vi "Autonomous Independent.vi"() -> ()   [LabVIEW 2017]
doc: "This VI is called when autonomous begins, and will automatically be terminated when autonomous ends. You can carry out timed or sensor driven robot movement independently without needing to return to the caller."
uses:
  CommandTypes/LiftCommands.ctl
  CommandTypes/AutoCommands.ctl
  <vilib>/Platform/TimedLoop/XDataNode/timing_clust.ctl
  <vilib>/Platform/TimedLoop/XDataNode/nitl_modes.ctl
  <vilib>/Platform/TimedLoop/XDataNode/wakeup.ctl
  <userlib>/836-Library/Drive/Drive_Code_V2/Drive_Code_Support/SensorTypedefs/Sensor_Cluster.ctl
  <userlib>/836-Library/Drive/Drive_Code_V2/Drive_Code_Support/SensorTypedefs/Camera_Cluster.ctl
  <vilib>/Rock Robotics/WPI/RobotDrive/WPI_RobotDriveDevRef.ctl
  <vilib>/Rock Robotics/WPI/MotorControl/WPI_MotorControlDeviceRef.ctl
  <vilib>/Rock Robotics/WPI/MotorControl/WPI_MotorControlType.ctl
  <vilib>/Rock Robotics/SystemInterfaces/DIO/FPGA_DIOPWMChannel.ctl
  <vilib>/Rock Robotics/WPI/PWM/WPI_PWMDeadband.ctl
  <vilib>/Rock Robotics/SystemInterfaces/DIO/FPGA_DIOChannel.ctl
  <userlib>/836-Library/Drive/Drive_Code_V2/Drive_Code_Support/DriveTrains/Drive_Trains.ctl
  <userlib>/836-Library/Drive/Drive_Code_V2/Drive_Code_Support/Command_Sends/Drive_Code_Command_Type.ctl
  <userlib>/836-Library/Drive/Drive_Code_V2/Drive_Code_Support/Command_Sends/Drive_Code_Command_List.ctl
  <userlib>/836-Library/Drive/Drive_Code_V2/Drive_Code_Support/PidClusters/PidInversions.ctl
  <userlib>/836-Library/Drive/Drive_Code_V2/Drive_Code_Support/PidClusters/DrivePidInputs.ctl
  <userlib>/836-Library/Drive/Drive_Code_V2/Drive_Code_Support/PidClusters/PidInputs.ctl
  <userlib>/836-Library/Drive/Drive_Code_V2/Drive_Code_Support/Command_Sends/Command_Tolerances.ctl
  <userlib>/836-Library/Drive/Drive_Code_V2/Drive_Code_Support/Command_Sends/Command_Tolerance_Info.ctl
  <userlib>/836-Library/Drive/Drive_Code_V2/Drive_Code_Support/CmdFinishedTypes.ctl
  CommandTypes/DriveCommands.ctl
  CommandTypes/IntakeCommands.ctl
  <vilib>/Rock Robotics/Network Tables/NT Read Number.vi
  <vilib>/Rock Robotics/Network Tables/NT Read Boolean.vi
  <vilib>/addons/control/pid/pid.llb/PID (DBL).vi
  <userlib>/836-Library/Drive/Drive_Code_V2/Drive_Code_Support/Command_Sends/Drive_Cmd_Cheesey_Drive.vi
  <userlib>/836-Library/Drive/Drive_Code_V2/Drive_Code_Support/Command_Sends/Drive_Cmd_Do_Nothing.vi
  <userlib>/836-Library/Drive/Drive_Code_V2/Drive_Code_Support/Command_Sends/Drive_Cmd_Drive_Distance.vi
  <vilib>/platform/TimedLoop/XDataNode/XDataNode.xnode
  <vilib>/Platform/TimedLoop/XDataNode/XDNodeRunTimeDep.lvlib
  <vilib>/addons/control/pid/NI_PID_pid.lvlib
  <userlib>/836-Library/Drive/Drive_Code_V2/Drive_Code_Support/Command_Sends/Drive_Cmd_Turn.vi
panel:
  in  "Y Points":dbl[](array[numeric])=[45.0, 40.0, 40.0, 45.0, 70.0]
  in  "X Points":dbl[](array[numeric])=[20.0, 50.0, 100.0, 200.0, 266.0]
  out "Throttle Cmd":dbl(graph)=-0.2211335616573206
  out "Steer Cmd":dbl(graph)=0.4174203899708857
  in  "Throttle Feed Fwd":dbl=0.28
  in  "Pid Setpoints":i32=500
  in  "Limit of Orientation Change":dbl=15.0 format="%#_13g"
  in  "Absolute Theta Final":dbl
  in  "Amount of Time (s)":dbl=4.0
  out "Steer Response":cluster{"setpoint":dbl, dbl}(graph)={"setpoint"=-0.6332041750032447, -21.50422367354753}
  in  "Steer Limit":cluster{"output high":dbl, "output low":dbl}={"output high"=0.5, "output low"=-0.5} {"output low" format="%.2f"; "output high" format="%.2f"}
  in  "Steer Gains":T1={"proportional gain (Kc)"=0.02, "integral time (Ti, min)"=0.0, "derivative time (Td, min)"=0.0} {"derivative time (Td, min)" format="%.3f"; "integral time (Ti, min)" format="%.3f"; "proportional gain (Kc)" format="%.3f"}
  out "Arc Response":cluster{"setpoint":dbl, dbl}(graph)={"setpoint"=251.75033529143298, 253.22199624999996}
  in  "Speed Limit":cluster{"output high":dbl, "output low":dbl}={"output high"=1.0, "output low"=-1.0} {"output low" format="%.2f"; "output high" format="%.2f"}
  in  "Speed Gains":T1={"proportional gain (Kc)"=0.04, "integral time (Ti, min)"=0.0, "derivative time (Td, min)"=0.0} {"derivative time (Td, min)" format="%.3f"; "integral time (Ti, min)" format="%.3f"; "proportional gain (Kc)" format="%.3f"}
  out "Auto Path Graph":cluster{"X":dbl, "Y":dbl}[](graph)=[{"X"=0.0, "Y"=0.0}, {"X"=0.29962072558749825, "Y"=0.0007367430518598614}, {"X"=0.5972966123215261, "Y"=0.0029335432231455886}, {"X"=0.8930518323738127, "Y"=0.0065702570374162475}, {"X"=1.1869105579160868, "Y"=0.011626741018230904}, {"X"=1.4788969611200782, "Y"=0.018082851689148624}, {"X"=1.7690352141575154, "Y"=0.025918445573728487}, {"X"=2.057349489200128, "Y"=0.035113379195529544}, {"X"=2.343863958419645, "Y"=0.04564750907811086}, {"X"=2.628602793987795, "Y"=0.057500691745031515}, {"X"=2.9115901680763074, "Y"=0.07065278371985056}, {"X"=3.192850252856912, "Y"=0.08508364152612709}, {"X"=3.4724072205013368, "Y"=0.10077312168742014}, {"X"=3.750285243181312, "Y"=0.1177010807272888}, {"X"=4.026508493068566, "Y"=0.13584737516929213}, {"X"=4.3011011423348275, "Y"=0.15519186153698913}, {"X"=4.574087363151827, "Y"=0.175714396353939}, {"X"=4.845491327691294, "Y"=0.19739483614370076}, {"X"=5.115337208124954, "Y"=0.2202130374298334}, {"X"=5.38364917662454, "Y"=0.24414885673589606}, {"X"=5.650451405361779, "Y"=0.2691821505854477}, {"X"=5.915768066508401, "Y"=0.2952927755020476}, {"X"=6.179623332236137, "Y"=0.3224605880092547}, {"X"=6.442041374716712, "Y"=0.35066544463062793}, {"X"=6.703046366121857, "Y"=0.37988720188972663}, {"X"=6.962662478623301, "Y"=0.4101057163101096}, {"X"=7.2209138843927745, "Y"=0.4413008444153362}, {"X"=7.477824755602007, "Y"=0.4734524427289652}, {"X"=7.733419264422724, "Y"=0.5065403677745559}, {"X"=7.987721583026658, "Y"=0.5405444760756672}, {"X"=8.240755883585535, "Y"=0.5754446241558583}, {"X"=8.492546338271088, "Y"=0.6112206685386881}, {"X"=8.743117119255043, "Y"=0.6478524657477159}, {"X"=8.992492398709132, "Y"=0.6853198723065006}, {"X"=9.24069634880508, "Y"=0.7236027447386013}, {"X"=9.48775314171462, "Y"=0.7626809395675768}, {"X"=9.73368694960948, "Y"=0.8025343133169868}, {"X"=9.978521944661388, "Y"=0.8431427225103897}, {"X"=10.222282299042075, "Y"=0.8844860236713451}, {"X"=10.464992184923267, "Y"=0.9265440733234118}, {"X"=10.706675774476695, "Y"=0.9692967279901487}, {"X"=10.94735723987409, "Y"=1.0127238441951152}, {"X"=11.187060753287179, "Y"=1.0568052784618704}, {"X"=11.425810486887691, "Y"=1.1015208873139732}, {"X"=11.663630612847356, "Y"=1.1468505272749825}, {"X"=11.900545303337903, "Y"=1.1927740548684576}, {"X"=12.13657873053106, "Y"=1.2392713266179574}, {"X"=12.371755066598556, "Y"=1.286322199047041}, {"X"=12.606098483712124, "Y"=1.333906528679268}, {"X"=12.839633154043486, "Y"=1.3820041720381968}, {"X"=13.072383249764378, "Y"=1.4305949856473863}, {"X"=13.304372943046527, "Y"=1.4796588260303962}, {"X"=13.535626406061661, "Y"=1.5291755497107853}, {"X"=13.76616781098151, "Y"=1.5791250132121126}, {"X"=13.996021329977804, "Y"=1.6294870730579374}, {"X"=14.225211135222267, "Y"=1.6802415857718185}, {"X"=14.453761398886636, "Y"=1.7313684078773153}, {"X"=14.681696293142636, "Y"=1.7828473958979865}, {"X"=14.909039990161995, "Y"=1.8346584063573912}, {"X"=15.135816662116438, "Y"=1.886781295779088}, {"X"=15.362050481177707, "Y"=1.9391959206866372}, {"X"=15.587765619517521, "Y"=1.9918821376035971}, {"X"=15.812986249307613, "Y"=2.0448198030535267}, {"X"=16.03773654271971, "Y"=2.097988773559986}, {"X"=16.26204067192554, "Y"=2.1513689056465326}, {"X"=16.485922809096838, "Y"=2.2049400558367265}, {"X"=16.709407126405328, "Y"=2.2586820806541263}, {"X"=16.93251779602274, "Y"=2.3125748366222916}, {"X"=17.155278990120802, "Y"=2.3665981802647806}, {"X"=17.377714880871245, "Y"=2.420731968105154}, {"X"=17.599849640445797, "Y"=2.474956056666968}, {"X"=17.82170744101619, "Y"=2.5292503024737854}, {"X"=18.04331245475415, "Y"=2.5835945620491625}, {"X"=18.26468885383141, "Y"=2.6379686919166594}, {"X"=18.48586081041969, "Y"=2.692352548599834}, {"X"=18.70685249669073, "Y"=2.7467259886222477}, {"X"=18.927688084816253, "Y"=2.8010688685074574}, {"X"=19.14839174696799, "Y"=2.855361044779024}, {"X"=19.36898765531767, "Y"=2.9095823739605042}, {"X"=19.589499982037022, "Y"=2.9637127125754597}, {"X"=19.809952899297773, "Y"=3.0177319171474464}, {"X"=20.030370579271654, "Y"=3.071619844200027}, {"X"=20.250777194130396, "Y"=3.125356350256758}, {"X"=20.471196916045724, "Y"=3.1789212918411995}, {"X"=20.691653917189374, "Y"=3.23229452547691}, {"X"=20.912172369733067, "Y"=3.28545590768745}, {"X"=21.132776445848535, "Y"=3.3383852949963764}, {"X"=21.35349031770751, "Y"=3.39106254392725}, {"X"=21.57433815748172, "Y"=3.4434675110036284}, {"X"=21.795344137342887, "Y"=3.495580052749072}, {"X"=22.01653242946275, "Y"=3.5473800256871395}, {"X"=22.237927206013033, "Y"=3.5988472863413894}, {"X"=22.459552639165466, "Y"=3.6499616912353807}, {"X"=22.68143290109178, "Y"=3.700703096892674}, {"X"=22.903592163963708, "Y"=3.7510513598368265}, {"X"=23.126054599952965, "Y"=3.800986336591399}, {"X"=23.34884438123129, "Y"=3.850487883679948}, {"X"=23.571985679970414, "Y"=3.8995358576260357}, {"X"=23.795502668342063, "Y"=3.9481101149532196}, {"X"=24.019419518517964, "Y"=3.9961905121850583}, {"X"=24.24376040266985, "Y"=4.043756905845111}, {"X"=24.468549492969448, "Y"=4.090789152456939}, {"X"=24.693810961588486, "Y"=4.137267108544098}, {"X"=24.9195689806987, "Y"=4.183170630630149}, {"X"=25.145847722471807, "Y"=4.22847957523865}, {"X"=25.37267135907955, "Y"=4.273173798893161}, {"X"=25.600064062693644, "Y"=4.317233158117241}, {"X"=25.828050005485824, "Y"=4.360637509434449}, {"X"=26.05665335962783, "Y"=4.403366709368345}, {"X"=26.28589829729137, "Y"=4.445400614442485}, {"X"=26.515808990648196, "Y"=4.486719081180431}, {"X"=26.746409611870018, "Y"=4.527301966105741}, {"X"=26.977724333128574, "Y"=4.567129125741975}, {"X"=27.209777326595592, "Y"=4.60618041661269}, {"X"=27.442592764442804, "Y"=4.644435695241447}, {"X"=27.676194818841932, "Y"=4.681874818151805}, {"X"=27.910607661964715, "Y"=4.718477641867323}, {"X"=28.145855465982866, "Y"=4.754224022911557}, {"X"=28.38196240306813, "Y"=4.7890938178080695}, {"X"=28.618952645392234, "Y"=4.82306688308042}, {"X"=28.8568503651269, "Y"=4.856123075252166}, {"X"=29.095679734443863, "Y"=4.888242250846866}, {"X"=29.335464925514845, "Y"=4.919404266388079}, {"X"=29.576230110511585, "Y"=4.949588978399366}, {"X"=29.817999461605805, "Y"=4.978776243404285}, {"X"=30.060797180862526, "Y"=5.006946007031386}, {"X"=30.30465108743448, "Y"=5.034088996613002}, {"X"=30.549596025396845, "Y"=5.06021687915411}, {"X"=30.795667645943535, "Y"=5.085343727494415}, {"X"=31.042901600268472, "Y"=5.109483614473622}, {"X"=31.291333539565585, "Y"=5.132650612931439}, {"X"=31.54099911502878, "Y"=5.154858795707567}, {"X"=31.79193397785199, "Y"=5.176122235641715}, {"X"=32.04417377922912, "Y"=5.196455005573586}, {"X"=32.29775417035411, "Y"=5.215871178342887}, {"X"=32.55271080242086, "Y"=5.234384826789322}, {"X"=32.809079326623305, "Y"=5.2520100237525975}, {"X"=33.06689539415536, "Y"=5.268760842072417}, {"X"=33.326194656210944, "Y"=5.284651354588488}, {"X"=33.58701276398397, "Y"=5.299695634140513}, {"X"=33.84938536866837, "Y"=5.3139077535682}, {"X"=34.11334812145807, "Y"=5.327301785711254}, {"X"=34.37893667354697, "Y"=5.339891803409379}, {"X"=34.646186676129005, "Y"=5.351691879502281}, {"X"=34.91513378039809, "Y"=5.362716086829666}, {"X"=35.18581363754814, "Y"=5.372978498231237}, {"X"=35.45826189877308, "Y"=5.382493186546703}, {"X"=35.73251421526684, "Y"=5.391274224615765}, {"X"=36.00860623822332, "Y"=5.399335685278132}, {"X"=36.28657361883646, "Y"=5.4066916413735076}, {"X"=36.56645200830016, "Y"=5.413356165741597}, {"X"=36.84827705780836, "Y"=5.419343331222105}, {"X"=37.132084418554975, "Y"=5.424667210654739}, {"X"=37.41790974173391, "Y"=5.429341876879203}, {"X"=37.70578867853911, "Y"=5.433381402735202}, {"X"=37.995756880164464, "Y"=5.436799861062442}, {"X"=38.287849997803924, "Y"=5.4396113247006275}, {"X"=38.58210368265139, "Y"=5.441829866489465}, {"X"=38.87855358590079, "Y"=5.443469559268658}, {"X"=39.177235358746046, "Y"=5.4445444758779145}, {"X"=39.47818465238106, "Y"=5.445068689156937}, {"X"=39.781437117999786, "Y"=5.4450562719454325}, {"X"=40.08702840679611, "Y"=5.444521297083106}, {"X"=40.39499416996397, "Y"=5.443477837409661}, {"X"=40.705370058697284, "Y"=5.441939965764806}, {"X"=41.018191724189975, "Y"=5.439921754988245}, {"X"=41.33349481763595, "Y"=5.437437277919683}, {"X"=41.651314990229146, "Y"=5.4345006073988245}, {"X"=41.97168789316346, "Y"=5.431125816265377}, {"X"=42.29464917763285, "Y"=5.427326977359043}, {"X"=42.620234494831195, "Y"=5.42311816351953}, {"X"=42.94847949595244, "Y"=5.418513447586543}, {"X"=43.279419832190506, "Y"=5.413526902399787}, {"X"=43.613091154739294, "Y"=5.408172600798967}, {"X"=43.949529114792746, "Y"=5.402464615623788}, {"X"=44.28876936354476, "Y"=5.396417019713956}, {"X"=44.63084755218928, "Y"=5.390043885909177}, {"X"=44.9757993319202, "Y"=5.383359287049155}, {"X"=45.32366035393147, "Y"=5.376377295973596}, {"X"=45.67446626941699, "Y"=5.3691119855222045}, {"X"=46.02825272957068, "Y"=5.361577428534686}, {"X"=46.38505538558647, "Y"=5.3537876978507475}, {"X"=46.74490988865826, "Y"=5.345756866310093}, {"X"=47.107851889980005, "Y"=5.337499006752427}, {"X"=47.47391704074559, "Y"=5.329028192017456}, {"X"=47.84314099214896, "Y"=5.320358494944885}, {"X"=48.21555939538402, "Y"=5.31150398837442}, {"X"=48.5912079016447, "Y"=5.3024787451457644}, {"X"=48.97012216212491, "Y"=5.293296838098625}, {"X"=49.352337828018584, "Y"=5.283972340072706}, {"X"=49.73789055051962, "Y"=5.2745193239077155}, {"X"=50.126815980821966, "Y"=5.264951862443355}, {"X"=50.519149770119526, "Y"=5.255284028519333}, {"X"=50.914927569606206, "Y"=5.245529894975353}, {"X"=51.31418503047596, "Y"=5.235703534651121}, {"X"=51.71695780392268, "Y"=5.225819020386341}, {"X"=52.1232815411403, "Y"=5.21589042502072}, {"X"=52.53319189332274, "Y"=5.205931821393963}, {"X"=52.946724511663916, "Y"=5.195957282345774}, {"X"=53.36391504735774, "Y"=5.185980880715861}, {"X"=53.78479915159815, "Y"=5.176016689343926}, {"X"=54.20941247557906, "Y"=5.166078781069676}, {"X"=54.63779067049438, "Y"=5.156181228732817}, {"X"=55.06996938753802, "Y"=5.1463381051730535}, {"X"=55.50598427790395, "Y"=5.136563483230091}, {"X"=55.94587099278605, "Y"=5.1268714357436345}, {"X"=56.38966518337824, "Y"=5.117276035553388}, {"X"=56.83740250087444, "Y"=5.10779135549906}, {"X"=57.2891185964686, "Y"=5.098431468420354}, {"X"=57.744849121354605, "Y"=5.089210447156975}, {"X"=58.204629726726395, "Y"=5.080142364548628}, {"X"=58.66849606377785, "Y"=5.07124129343502}, {"X"=59.136483783702964, "Y"=5.062521306655855}, {"X"=59.6086285376956, "Y"=5.0539964770508385}, {"X"=60.08496597694969, "Y"=5.045680877459676}, {"X"=60.56553175265917, "Y"=5.0375885807220735}, {"X"=61.050361516017944, "Y"=5.029733659677735}, {"X"=61.53949091821995, "Y"=5.022130187166366}, {"X"=62.03295561045906, "Y"=5.014792236027673}, {"X"=62.53079124392925, "Y"=5.007733879101359}, {"X"=63.03303346982443, "Y"=5.000969189227131}, {"X"=63.53971793933851, "Y"=4.9945122392446955}, {"X"=64.05088030366538, "Y"=4.9883771019937555}, {"X"=64.56655621399901, "Y"=4.982577850314018}, {"X"=65.08678132153331, "Y"=4.977128557045186}, {"X"=65.61159127746217, "Y"=4.972043295026968}, {"X"=66.14102173297954, "Y"=4.967336137099067}, {"X"=66.67510833927932, "Y"=4.963021156101189}, {"X"=67.21388674755546, "Y"=4.959112424873039}, {"X"=67.75739260900183, "Y"=4.955624016254323}, {"X"=68.3056615748124, "Y"=4.952570003084746}, {"X"=68.85872929618108, "Y"=4.949964458204013}, {"X"=69.41663142430178, "Y"=4.947821454451829}, {"X"=69.9794036103684, "Y"=4.946155064667901}, {"X"=70.54708150557488, "Y"=4.9449793616919315}, {"X"=71.11970076111515, "Y"=4.944308418363629}, {"X"=71.69729702818313, "Y"=4.944156307522697}, {"X"=72.27990595797272, "Y"=4.94453710200884}, {"X"=72.86756320167787, "Y"=4.945464874661765}, {"X"=73.46030441049247, "Y"=4.946953698321177}, {"X"=74.05816523561043, "Y"=4.949017645826781}, {"X"=74.66118132822572, "Y"=4.951670790018282}, {"X"=75.26938833953223, "Y"=4.954927203735385}, {"X"=75.88282192072388, "Y"=4.958800959817797}, {"X"=76.50151772299456, "Y"=4.963306131105221}, {"X"=77.12551139753825, "Y"=4.968456790437365}, {"X"=77.75483859554886, "Y"=4.974267010653931}, {"X"=78.38953496822026, "Y"=4.980750864594628}, {"X"=79.02963616674641, "Y"=4.987922425099159}, {"X"=79.67517784232123, "Y"=4.995795765007229}, {"X"=80.32619336045194, "Y"=5.004383910893502}, {"X"=80.98266351585136, "Y"=5.013675825236637}, {"X"=81.64451653243808, "Y"=5.0236364064193015}, {"X"=82.3116783484439, "Y"=5.034229506559112}, {"X"=82.98407490210067, "Y"=5.045418977773689}, {"X"=83.66163213164016, "Y"=5.057168672180652}, {"X"=84.34427597529427, "Y"=5.069442441897622}, {"X"=85.03193237129477, "Y"=5.082204139042218}, {"X"=85.72452725787349, "Y"=5.0954176157320585}, {"X"=86.42198657326229, "Y"=5.109046724084765}, {"X"=87.12423625569298, "Y"=5.123055316217956}, {"X"=87.83120224339737, "Y"=5.137407244249251}, {"X"=88.54281047460726, "Y"=5.15206636029627}, {"X"=89.25898688755456, "Y"=5.166996516476634}, {"X"=89.97965742047104, "Y"=5.182161564907961}, {"X"=90.70474801158852, "Y"=5.197525357707872}, {"X"=91.43418459913882, "Y"=5.213051746993985}, {"X"=92.1678931213538, "Y"=5.228704584883921}, {"X"=92.90579951646528, "Y"=5.2444477234953}, {"X"=93.64782972270503, "Y"=5.26024501494574}, {"X"=94.39390967830495, "Y"=5.276060311352863}, {"X"=95.14396532149684, "Y"=5.291857464834287}, {"X"=95.89792259051252, "Y"=5.307600327507632}, {"X"=96.65570742358378, "Y"=5.323252751490518}, {"X"=97.4172457589425, "Y"=5.338778588900565}, {"X"=98.1824635348205, "Y"=5.354141691855392}, {"X"=98.95128668944957, "Y"=5.369305912472619}, {"X"=99.72364116106155, "Y"=5.384235102869865}, {"X"=100.49945288788828, "Y"=5.398893115164751}, {"X"=101.2786478081616, "Y"=5.413243801474897}, {"X"=102.06115186011326, "Y"=5.427251013917919}, {"X"=102.84689098197518, "Y"=5.4408786046114415}, {"X"=103.63579111197913, "Y"=5.454090425673082}, {"X"=104.42777818835697, "Y"=5.466850329220461}, {"X"=105.22277814934046, "Y"=5.479122167371195}, {"X"=106.0207169331615, "Y"=5.490869792242909}, {"X"=106.82152047805188, "Y"=5.502057055953219}, {"X"=107.62511472224344, "Y"=5.512647810619745}, {"X"=108.43142560396794, "Y"=5.522605908360108}, {"X"=109.24037906145732, "Y"=5.531895201291926}, {"X"=110.05190103294333, "Y"=5.540479541532821}, {"X"=110.86591745665778, "Y"=5.54832278120041}, {"X"=111.68235427083256, "Y"=5.555388772412315}, {"X"=112.50113741369947, "Y"=5.561641367286155}, {"X"=113.32219282349033, "Y"=5.567044417939549}, {"X"=114.1454464384369, "Y"=5.571561776490117}, {"X"=114.97082419677113, "Y"=5.5751572950554795}, {"X"=115.79825203672479, "Y"=5.577794825753255}, {"X"=116.62765589652966, "Y"=5.579438220701063}, {"X"=117.4589617144176, "Y"=5.5800513320165255}, {"X"=118.29209542862048, "Y"=5.57959801181726}, {"X"=119.12698297737006, "Y"=5.578042112220887}, {"X"=119.96355029889817, "Y"=5.575347485345026}, {"X"=120.8017233314367, "Y"=5.571477983307297}, {"X"=121.64142801321742, "Y"=5.566397458225318}, {"X"=122.48259028247216, "Y"=5.5600697622167115}, {"X"=123.32513607743273, "Y"=5.552458747399096}, {"X"=124.168991336331, "Y"=5.543528265890091}, {"X"=125.01408199739879, "Y"=5.533242169807315}, {"X"=125.8603339988679, "Y"=5.521564311268389}, {"X"=126.70767327897012, "Y"=5.508458542390934}, {"X"=127.55602577593737, "Y"=5.4938887152925675}, {"X"=128.4053174280014, "Y"=5.47781868209091}, {"X"=129.25547417339405, "Y"=5.460212294903582}, {"X"=130.10642195034717, "Y"=5.441033405848201}, {"X"=130.9580866970926, "Y"=5.4202458670423885}, {"X"=131.8103943518621, "Y"=5.397813530603764}, {"X"=132.6632708528875, "Y"=5.373700248649947}, {"X"=133.51664213840073, "Y"=5.347869873298557}, {"X"=134.3704341466335, "Y"=5.320286256667213}, {"X"=135.22457281581768, "Y"=5.290913250873538}, {"X"=136.0789840841851, "Y"=5.259714708035148}, {"X"=136.9335938899676, "Y"=5.226654480269662}, {"X"=137.78832817139696, "Y"=5.191696419694703}, {"X"=138.643112866705, "Y"=5.154804378427891}, {"X"=139.4978739141236, "Y"=5.115942208586842}, {"X"=140.35253725188457, "Y"=5.075073762289178}, {"X"=141.20702881821973, "Y"=5.0321628916525185}, {"X"=142.06127455136087, "Y"=4.9871734487944845}, {"X"=142.91520038953985, "Y"=4.940069285832693}, {"X"=143.76873227098855, "Y"=4.890814254884764}, {"X"=144.62179613393863, "Y"=4.839372208068322}, {"X"=145.4743179166221, "Y"=4.785706997500979}, {"X"=146.3262235572707, "Y"=4.729782475300358}, {"X"=147.17743899411627, "Y"=4.671562493584082}, {"X"=148.0278901653906, "Y"=4.611010904469768}, {"X"=148.87750300932555, "Y"=4.548091560075034}, {"X"=149.72620346415295, "Y"=4.482768312517502}, {"X"=150.57391746810464, "Y"=4.41500501391479}, {"X"=151.42057095941237, "Y"=4.344765516384522}, {"X"=152.26608987630803, "Y"=4.272013672044311}, {"X"=153.11040015702346, "Y"=4.196713333011781}, {"X"=153.9534277397904, "Y"=4.118828351404554}, {"X"=154.79509856284076, "Y"=4.038322579340243}, {"X"=155.63533856440637, "Y"=3.955159868936471}, {"X"=156.474073682719, "Y"=3.8693040723108583}, {"X"=157.31122985601047, "Y"=3.7807190415810275}, {"X"=158.14673302251265, "Y"=3.689368628864591}, {"X"=158.98050912045738, "Y"=3.5952166862791737}, {"X"=159.81248408807642, "Y"=3.498227065942393}, {"X"=160.6425838636016, "Y"=3.3983636199718736}, {"X"=161.47073438526482, "Y"=3.295590200485228}, {"X"=162.29686159129787, "Y"=3.1898706596000785}, {"X"=163.12089141993252, "Y"=3.081168849434051}, {"X"=163.94274980940065, "Y"=2.969448622104754}, {"X"=164.76236269793412, "Y"=2.854673829729813}, {"X"=165.5796560237647, "Y"=2.7368083244268484}, {"X"=166.39455572512418, "Y"=2.615815958313483}, {"X"=167.20698774024447, "Y"=2.4916605835073273}, {"X"=168.01687800735735, "Y"=2.364306052126008}, {"X"=168.8241524646947, "Y"=2.233716216287141}, {"X"=169.6287370504882, "Y"=2.0998549281083543}, {"X"=170.43055770296985, "Y"=1.9626860397072563}, {"X"=171.22954036037137, "Y"=1.8221734032014707}, {"X"=172.0256109609246, "Y"=1.6782808707086256}, {"X"=172.81869544286138, "Y"=1.5309722943463262}, {"X"=173.60871974441358, "Y"=1.3802115262321992}, {"X"=174.395609803813, "Y"=1.225962418483865}, {"X"=175.17929155929136, "Y"=1.0681888232189483}, {"X"=175.9596909490806, "Y"=0.9068545925550575}, {"X"=176.73673391141256, "Y"=0.7419235786098177}, {"X"=177.51034638451898, "Y"=0.5733596335008491}, {"X"=178.28045430663173, "Y"=0.40112660934577704}, {"X"=179.04698361598264, "Y"=0.22518835826221117}, {"X"=179.80986025080355, "Y"=0.04550873236777253}, {"X"=180.5690154266411, "Y"=-0.1379399569945681}, {"X"=181.32442629122727, "Y"=-0.32511177189097307}, {"X"=182.0760936424828, "Y"=-0.5159228645258761}, {"X"=182.8240184737846, "Y"=-0.7102890737990789}, {"X"=183.5682017785096, "Y"=-0.9081262386103742}, {"X"=184.30864455003476, "Y"=-1.1093501978595812}, {"X"=185.04534778173695, "Y"=-1.3138767904464923}, {"X"=185.77831246699316, "Y"=-1.5216218552709098}, {"X"=186.50753959918018, "Y"=-1.7325012312326256}, {"X"=187.23303017167507, "Y"=-1.9464307572314596}, {"X"=187.95478517785472, "Y"=-2.163326272167204}, {"X"=188.67280561109595, "Y"=-2.383103614939652}, {"X"=189.3870924647758, "Y"=-2.6056786244486227}, {"X"=190.09764673227116, "Y"=-2.830967139593909}, {"X"=190.8044694069589, "Y"=-3.0588849992753127}, {"X"=191.50756148221598, "Y"=-3.289348042392625}, {"X"=192.20692395141933, "Y"=-3.522272107845667}, {"X"=192.90255780794587, "Y"=-3.7575730345342313}, {"X"=193.5944640451725, "Y"=-3.9951666613581187}, {"X"=194.28264365647613, "Y"=-4.234968827217121}, {"X"=194.9670976352337, "Y"=-4.47689537101106}, {"X"=195.64782697482215, "Y"=-4.720862131639728}, {"X"=196.32483266861834, "Y"=-4.966784948002913}, {"X"=196.99811570999924, "Y"=-5.214579659000441}, {"X"=197.6676770923418, "Y"=-5.464162103532102}, {"X"=198.33351780902285, "Y"=-5.715448120497686}, {"X"=198.99563885341936, "Y"=-5.968353548797018}, {"X"=199.65404121890828, "Y"=-6.222794227329887}, {"X"=200.3087258988665, "Y"=-6.478685994996095}, {"X"=200.95969388667095, "Y"=-6.735944690695444}, {"X"=201.6069461756985, "Y"=-6.994486153327736}, {"X"=202.2504837593261, "Y"=-7.254226221792747}, {"X"=202.89030763093075, "Y"=-7.5150807349903275}, {"X"=203.52641878388926, "Y"=-7.776965531820255}, {"X"=204.15881821157862, "Y"=-8.039796451182331}, {"X"=204.7875069073757, "Y"=-8.303489331976358}, {"X"=205.41248586465747, "Y"=-8.567960013102136}, {"X"=206.0337560768008, "Y"=-8.833124333459468}, {"X"=206.65131853718265, "Y"=-9.098898131948154}, {"X"=207.26517423917986, "Y"=-9.365197247467975}, {"X"=207.87532417616947, "Y"=-9.631937518918777}, {"X"=208.48176934152835, "Y"=-9.899034785200337}, {"X"=209.08451072863343, "Y"=-10.16640488521246}, {"X"=209.6835493308616, "Y"=-10.433963657854944}, {"X"=210.2788861415898, "Y"=-10.701626942027595}, {"X"=210.87052215419493, "Y"=-10.969310576630209}, {"X"=211.4584583620539, "Y"=-11.236930400562569}, {"X"=212.04269575854372, "Y"=-11.504402252724521}, {"X"=212.62323533704122, "Y"=-11.771641972015846}, {"X"=213.20007809092334, "Y"=-12.03856539733634}, {"X"=213.77322501356704, "Y"=-12.30508836758581}, {"X"=214.3426770983492, "Y"=-12.571126721664054}, {"X"=214.90843533864674, "Y"=-12.836596298470877}, {"X"=215.47050072783657, "Y"=-13.101412936906053}, {"X"=216.02887425929563, "Y"=-13.365492475869434}, {"X"=216.5835569264009, "Y"=-13.628750754260796}, {"X"=217.1345497225292, "Y"=-13.891103610979942}, {"X"=217.6818536410575, "Y"=-14.152466884926673}, {"X"=218.2254696753627, "Y"=-14.412756415000791}, {"X"=218.76539881882172, "Y"=-14.671888040102095}, {"X"=219.30164206481155, "Y"=-14.929777599130391}, {"X"=219.83420040670896, "Y"=-15.186340930985457}, {"X"=220.36307483789102, "Y"=-15.441493874567135}, {"X"=220.8882663517346, "Y"=-15.69515226877521}, {"X"=221.4097759416166, "Y"=-15.94723195250948}, {"X"=221.92760460091398, "Y"=-16.197648764669747}, {"X"=222.4417533230036, "Y"=-16.44631854415581}, {"X"=222.95222310126246, "Y"=-16.69315712986748}, {"X"=223.45901492906737, "Y"=-16.93808036070453}, {"X"=223.96212979979535, "Y"=-17.1810040755668}, {"X"=224.4615687068233, "Y"=-17.421844113354084}, {"X"=224.9573326435281, "Y"=-17.660516312966166}, {"X"=225.44942260328673, "Y"=-17.89693651330286}, {"X"=225.93783957947605, "Y"=-18.131020553263966}, {"X"=226.42258456547302, "Y"=-18.362684271749284}, {"X"=226.90365855465453, "Y"=-18.591843507658595}, {"X"=227.38106254039752, "Y"=-18.818414099891736}, {"X"=227.85479751607895, "Y"=-19.0423118873485}, {"X"=228.32486447507566, "Y"=-19.263452708928682}, {"X"=228.79126441076463, "Y"=-19.48175240353208}, {"X"=229.25399831652277, "Y"=-19.697126810058503}, {"X"=229.71306718572697, "Y"=-19.909491767407747}, {"X"=230.16847201175418, "Y"=-20.118763114479613}, {"X"=230.62021378798127, "Y"=-20.32485669017389}, {"X"=231.06829350778526, "Y"=-20.52768833339041}, {"X"=231.51271216454296, "Y"=-20.727173883028964}, {"X"=231.9534707516314, "Y"=-20.923229177989345}, {"X"=232.39057026242742, "Y"=-21.115770057171357}, {"X"=232.82401169030794, "Y"=-21.304712359474806}, {"X"=233.25379602864996, "Y"=-21.489971923799487}, {"X"=233.67992427083027, "Y"=-21.671464589045197}, {"X"=234.10239741022588, "Y"=-21.84910619411175}, {"X"=234.52121644021372, "Y"=-22.022812577898954}, {"X"=234.9363823541707, "Y"=-22.192499579306592}, {"X"=235.3478961454737, "Y"=-22.35808303723448}, {"X"=235.75575880749966, "Y"=-22.519478790582408}, {"X"=236.15997133362552, "Y"=-22.676602678250187}, {"X"=236.56053471722817, "Y"=-22.829370539137596}, {"X"=236.95744995168457, "Y"=-22.977698212144468}, {"X"=237.35071803037158, "Y"=-23.121501536170594}, {"X"=237.7403399466662, "Y"=-23.260696350115776}, {"X"=238.1263166939453, "Y"=-23.395198492879803}, {"X"=238.5086492655858, "Y"=-23.524923803362494}, {"X"=238.88733865496465, "Y"=-23.64978812046364}, {"X"=239.26238585545872, "Y"=-23.769707283083047}, {"X"=239.63379186044494, "Y"=-23.884597130120504}, {"X"=240.0015576633003, "Y"=-23.99437350047583}, {"X"=240.36568425740165, "Y"=-24.098952233048824}, {"X"=240.72617263612594, "Y"=-24.198249166739277}, {"X"=241.08302379285007, "Y"=-24.292180140447005}, {"X"=241.43623872095097, "Y"=-24.3806609930718}, {"X"=241.78581841380557, "Y"=-24.463607563513463}, {"X"=242.13176386479074, "Y"=-24.54093569067179}, {"X"=242.4740760672835, "Y"=-24.6125612134466}, {"X"=242.8127560146607, "Y"=-24.678399970737686}, {"X"=243.14780470029928, "Y"=-24.738367801444845}, {"X"=243.4792231175761, "Y"=-24.79238054446789}, {"X"=243.8070122598682, "Y"=-24.840354038706604}, {"X"=244.1311731205524, "Y"=-24.882204123060802}, {"X"=244.45170669300563, "Y"=-24.917846636430284}, {"X"=244.7686139706049, "Y"=-24.947197417714847}, {"X"=245.081895946727, "Y"=-24.9701723058143}, {"X"=245.39155361474897, "Y"=-24.98668713962844}, {"X"=245.69758796804766, "Y"=-24.99665775805707}, {"X"=246.0, "Y"=-24.999999999999993}]
  out "Init Heights Queue":T2[](array[typedef])
  out "Init Turns Queue":dbl[](array[numeric])
  out "Init Points Queue":cluster{"X Points":dbl[], "Y Points":dbl[]}[](array[cluster])
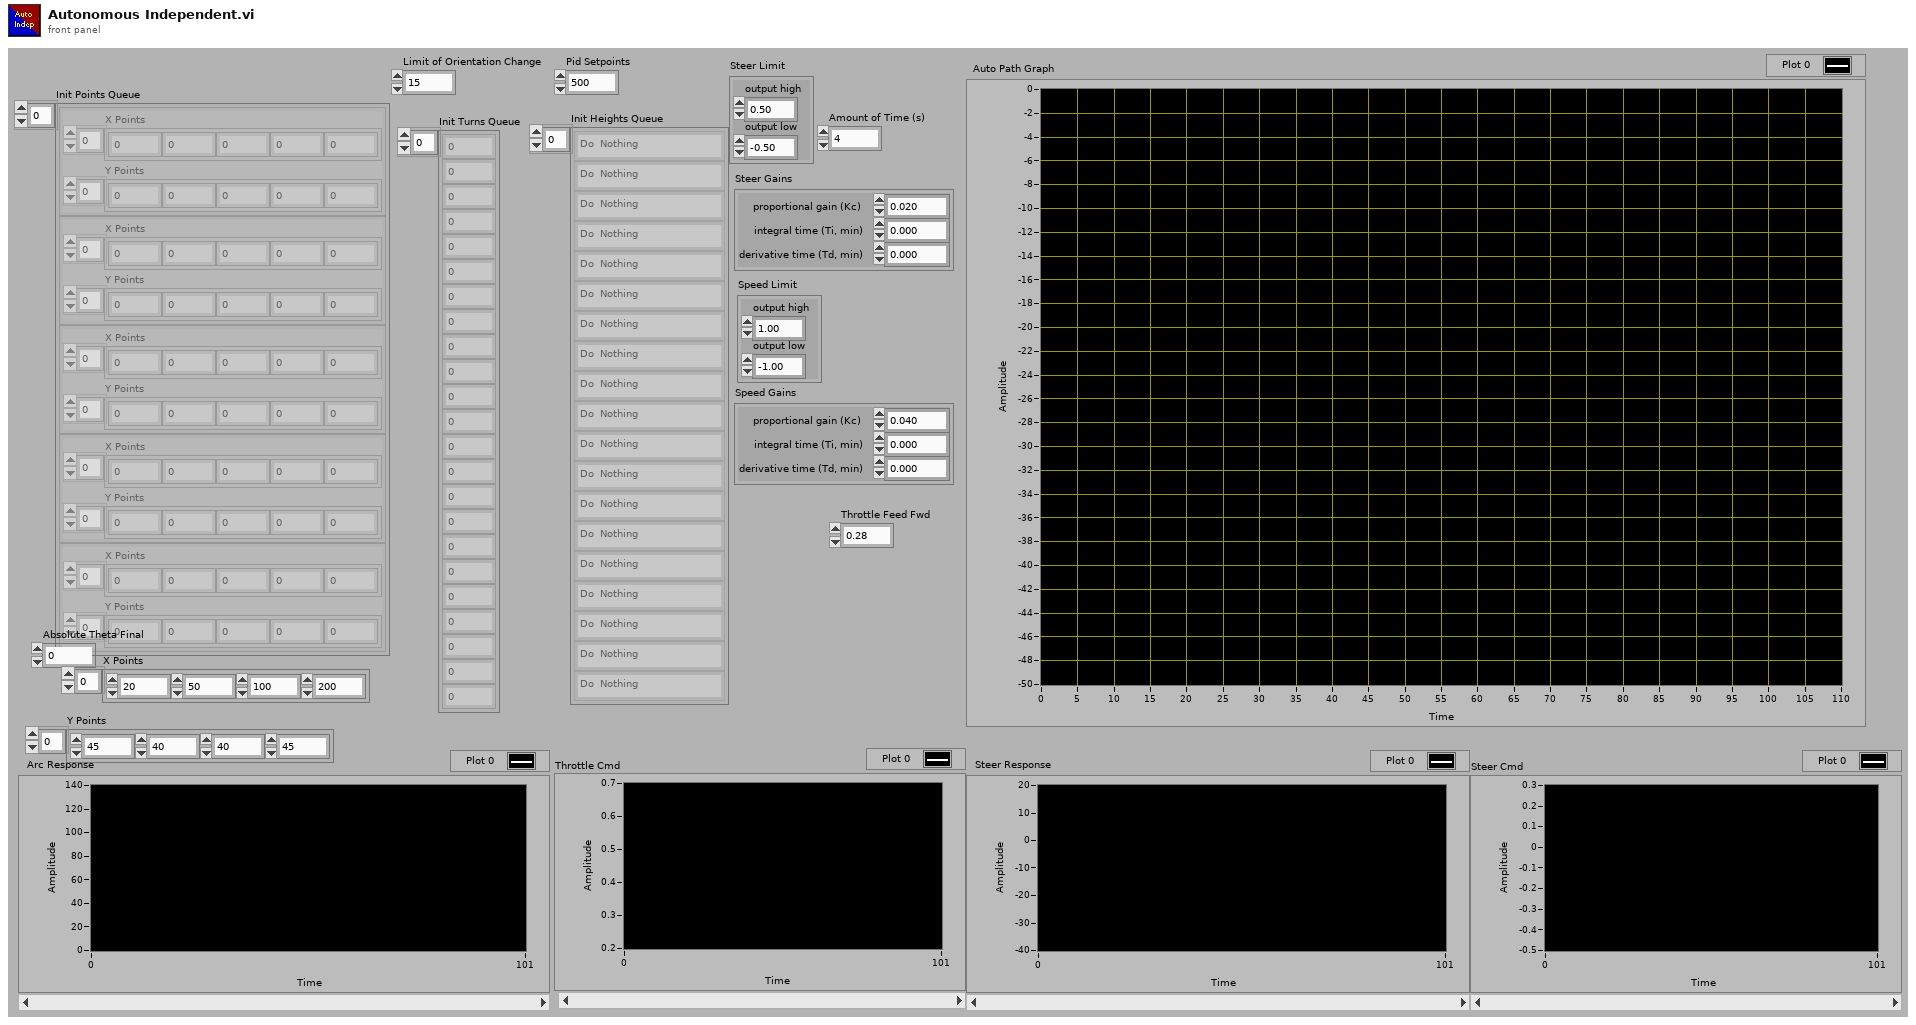
[diagram p1: front panel]
types:
  T1 = cluster{"proportional gain (Kc)":dbl, "integral time (Ti, min)":dbl, "derivative time (Td, min)":dbl}
  T2 = typedef "LiftCommands.ctl" = enum16{"Do  Nothing", "Manuel", "Ground", "Home", "To Switch", "To Scale Low", "To Scale Medium", "To Scale High"}
  T3 = typedef "AutoCommands.ctl" = enum16{"Delay", "Send Drive Command", "Move Lift", "Turn In Place", "Acquire Cube", "Score Cube", "Do Nothing", "Drive Straight"}
  T4 = typedef "XDNodeRunTimeDep.lvlib/timing_clust.ctl" = cluster{"Expected End [f-1]":u64, "Actual End [f-1]":u64, "Finished Late? [f-1]":bool, "Expected End [i-1]":u64, "Actual End [i-1]":u64, "Finished Late? [i-1]":bool, "Expected Start [i]":u64, "Actual Start [i]":u64, "Expected Start [f]":u64, "Actual Start [f]":u64, "Source Name":string, "Structure Name":string, "Period":i64, "Deadline":i64, "Offset":i64, "Start":i64, "Priority":i32, "Timeout":i32, "Mode":T5, "Wakeup Reason":T6, "Error":errorcluster, "Source Type":string, "Secondary Source Type":string, "Global End Time":u64, "Global Start Time":u64, "Frame Duration":u64, "Iteration Duration":u64, "Assigned CPU":i32, "I/O Scan Engine Mode":u32}
  T5 = typedef "XDNodeRunTimeDep.lvlib/nitl_modes.ctl" = enum32{"No Change", "Process missed periods, maintain original phase", "Discard missed periods, maintain original phase", "Process missed periods, ignore original phase", "Discard missed periods, ignore original phase"}
  T6 = typedef "XDNodeRunTimeDep.lvlib/wakeup.ctl" = enum32{"Normal", "Aborted", "Asynchronous wakeup", "Timing source error", "Timed loop error", "Timeout"}
  T7 = cluster{"Absolute Theta initial":dbl, "Absolute Theta Final":dbl}
  T8 = typedef "CmdFinishedTypes.ctl" = enum16{"Poll", "Blocking"}
  T9 = typedef "DriveCommands.ctl" = enum16{"Center on Cube", "Manual", "Acquire Cube", "Drive Path"}
  T10 = typedef "IntakeCommands.ctl" = enum16{"Do Nothing", "Manuel", "Score", "Acquire"}
  T11 = typedef "Command_Tolerances.ctl" = cluster{"Distance":T12, "Yaw":T12}
  T12 = typedef "Command_Tolerance_Info.ctl" = cluster{"Upper Error Bound":dbl, "Lower Error Bound":dbl}
  T13 = typedef "KeyPoints.ctl" = enum16{"Start_1", "Start_2", "Start_3", "Switch_L", "Switch_R", "Scale_L", "Scale_R", "Cube_1", "Cube_2", "Cube_3", "Cube_4", "Cube_5", "Cube_6", "CubeAcq_L", "CubeAcq_R", "Switch_Back_L", "Switch_Back_R"}
  T14 = typedef "Sensor_Cluster.ctl" = cluster{"Gyro Data":cluster{"Gyro RT FIFO":refnum<k33>, "Gyro Current":dbl, "Gyro Hold":dbl}, "Encoder Data":cluster{"Encoder RT FIFO":refnum<k33>, "Encoder Current":dbl, "Encoder Hold":dbl}, "Camera Data":cluster{"Camera RT FIFO":refnum<k33>, "Camera Current":T15}}
  T15 = typedef "Camera_Cluster.ctl" = cluster{" Angle":dbl, "Valid":bool}
  T16 = typedef "WPI_RobotDriveDevRef.ctl" = cluster{"DevStatus":errorcluster, "Motors[]":T17[], "Square Inputs":bool, "Max Output":dbl}
  T17 = typedef "WPI_MotorControlDeviceRef.ctl" = cluster{"DeviceStatus":errorcluster, "Type":T18, "PWM":cluster{"PWM Channel":T19, "DeadBand":T20}, "CAN":cluster{"Device Number":u8, "SetOutput VI Ref":variant, "GetOutput VI Ref":variant, "Enable VI Ref":variant, "Disable VI Ref":variant, "Data":variant}, "Invert":bool, "DIO PWM":cluster{"PWM \"Enable\" Channel":T19, "DIOChannel":T21, "PWM Rate":dbl}}
  T18 = typedef "WPI_MotorControlType.ctl" = enum16{"PWM", "CAN", "DIO PWM"}
  T19 = typedef "FPGA_DIOPWMChannel.ctl" = enum8{"PWM 0", "PWM 1", "PWM 2", "PWM 3", "PWM 4", "PWM 5", "PWM 6", "PWM 7", "PWM 8", "PWM 9", "PWM MXP 0", "PWM MXP 1", "PWM MXP 2", "PWM MXP 3", "PWM MXP 4", "PWM MXP 5", "PWM MXP 6", "PWM MXP 7", "PWM MXP 8", "PWM MXP 9", "Invalid"}
  T20 = typedef "WPI_PWMDeadband.ctl" = cluster{"Name":string, "maxPositivePwm":i32, "minPositivePwm":i32, "centerPwm":i32, "maxNegativePwm":i32, "minNegativePwm":i32, "angularRange":u16}
  T21 = typedef "FPGA_DIOChannel.ctl" = enum8{"DIO 0", "DIO 1", "DIO 2", "DIO 3", "DIO 4", "DIO 5", "DIO 6", "DIO 7", "DIO 8", "DIO 9", "DIO MXP 0", "DIO MXP 1", "DIO MXP 2", "DIO MXP 3", "DIO MXP 4", "DIO MXP 5", "DIO MXP 6", "DIO MXP 7", "DIO MXP 8", "DIO MXP 9", "DIO MXP 10", "DIO MXP 11", "DIO MXP 12", "DIO MXP 13", "DIO MXP 14", "DIO MXP 15", "SPI Port CS1", "SPI Port CS2", "SPI Port CS3", "SPI Port MISO", "SPI Port MOSI", "Invalid"}
  T22 = typedef "Drive_Trains.ctl" = enum16{"Tank Drive 2 Motor", "Tank Drive 4 Motor", "Tank Drive 6 Motor", "Mecanum Drive", "Kiwi Drive", "Invalid"}
  T23 = typedef "PidInversions.ctl" = cluster{"Distance PID Inverted?":bool, "Yaw PID Inverted?":bool}
  T24 = cluster{"Cluster":T14, "RobotDriveDevRef":T16, "Enum":T22, "Valid Commands":bool[], "Drive Comand Notifier":refnum<notifier>, "Command Finished?":refnum<k4>, "Command Canceled":refnum<k4>, "PID Inversions":T23, "PID Inputs Notifier":refnum<notifier>, "Cmd Tol Notifier":refnum<notifier>}
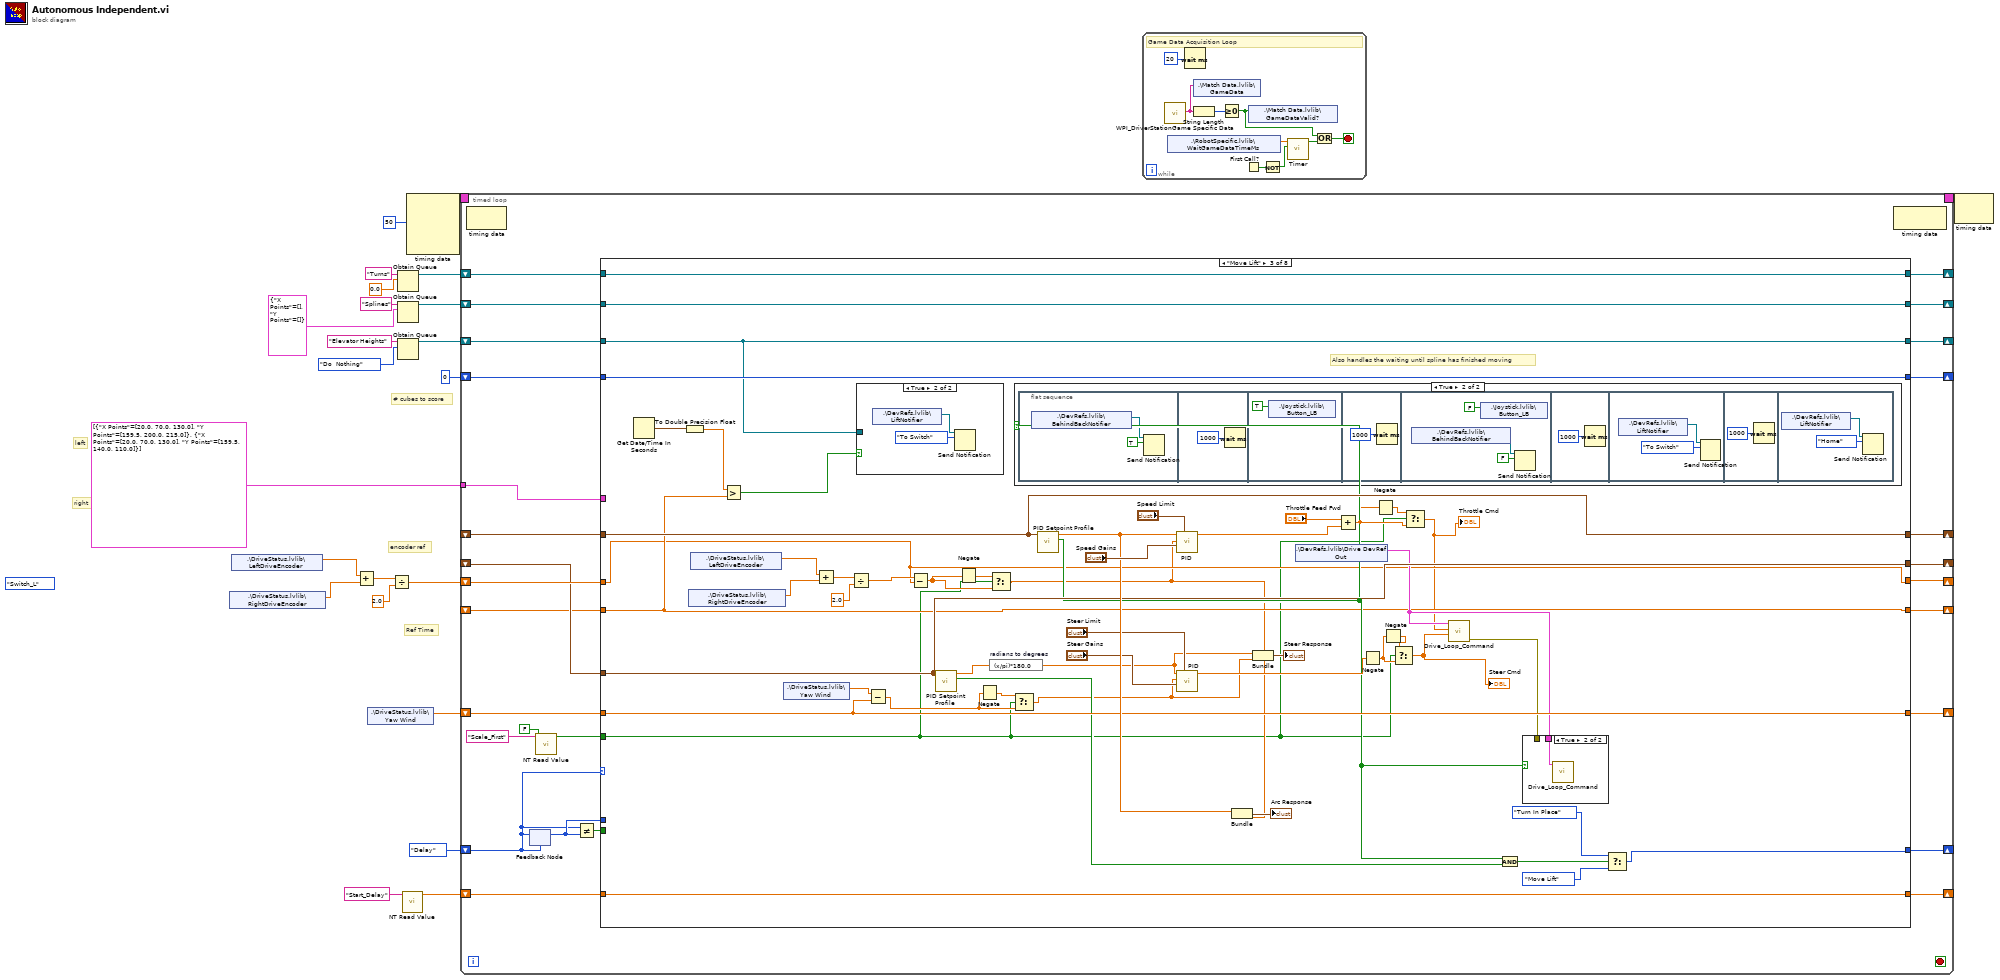
[diagram p0: block diagram]
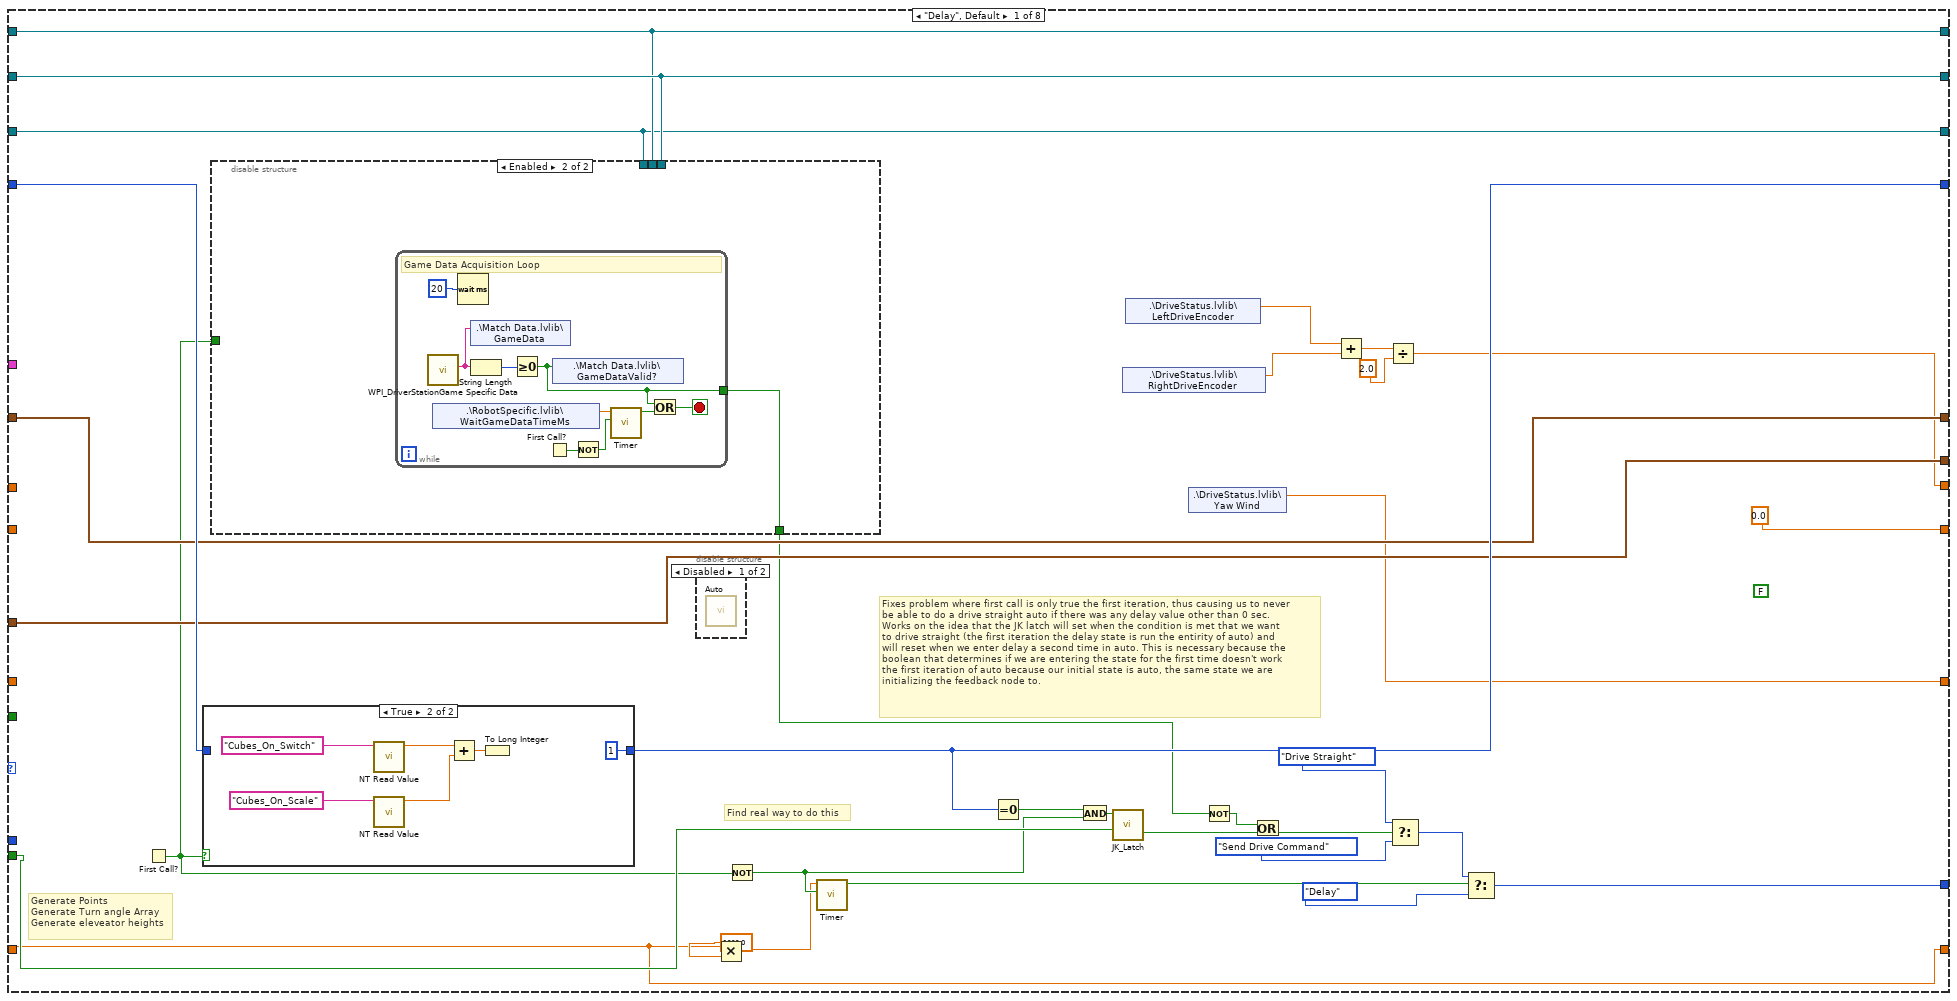
[diagram p2: hidden frame]
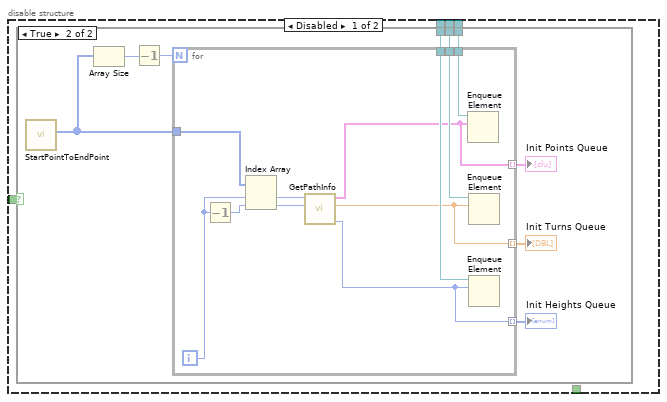
[diagram p3: hidden frame]
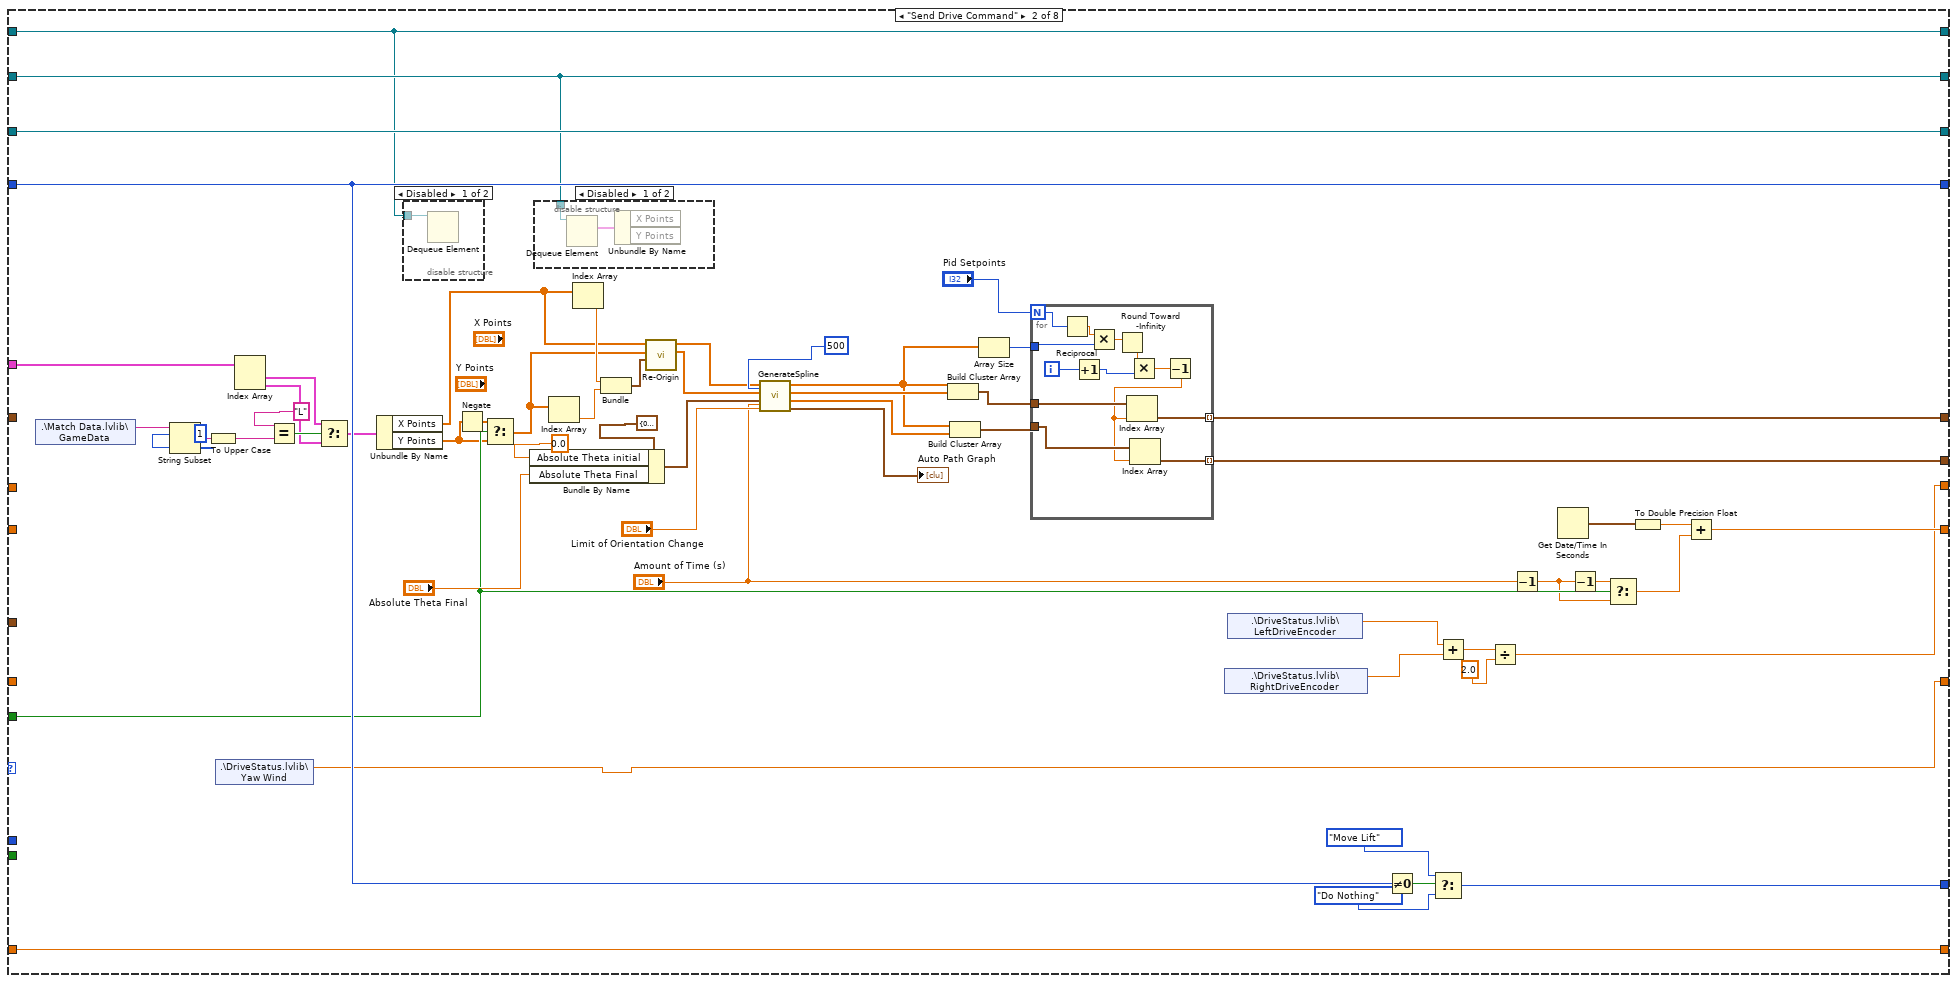
[diagram p7: hidden frame]
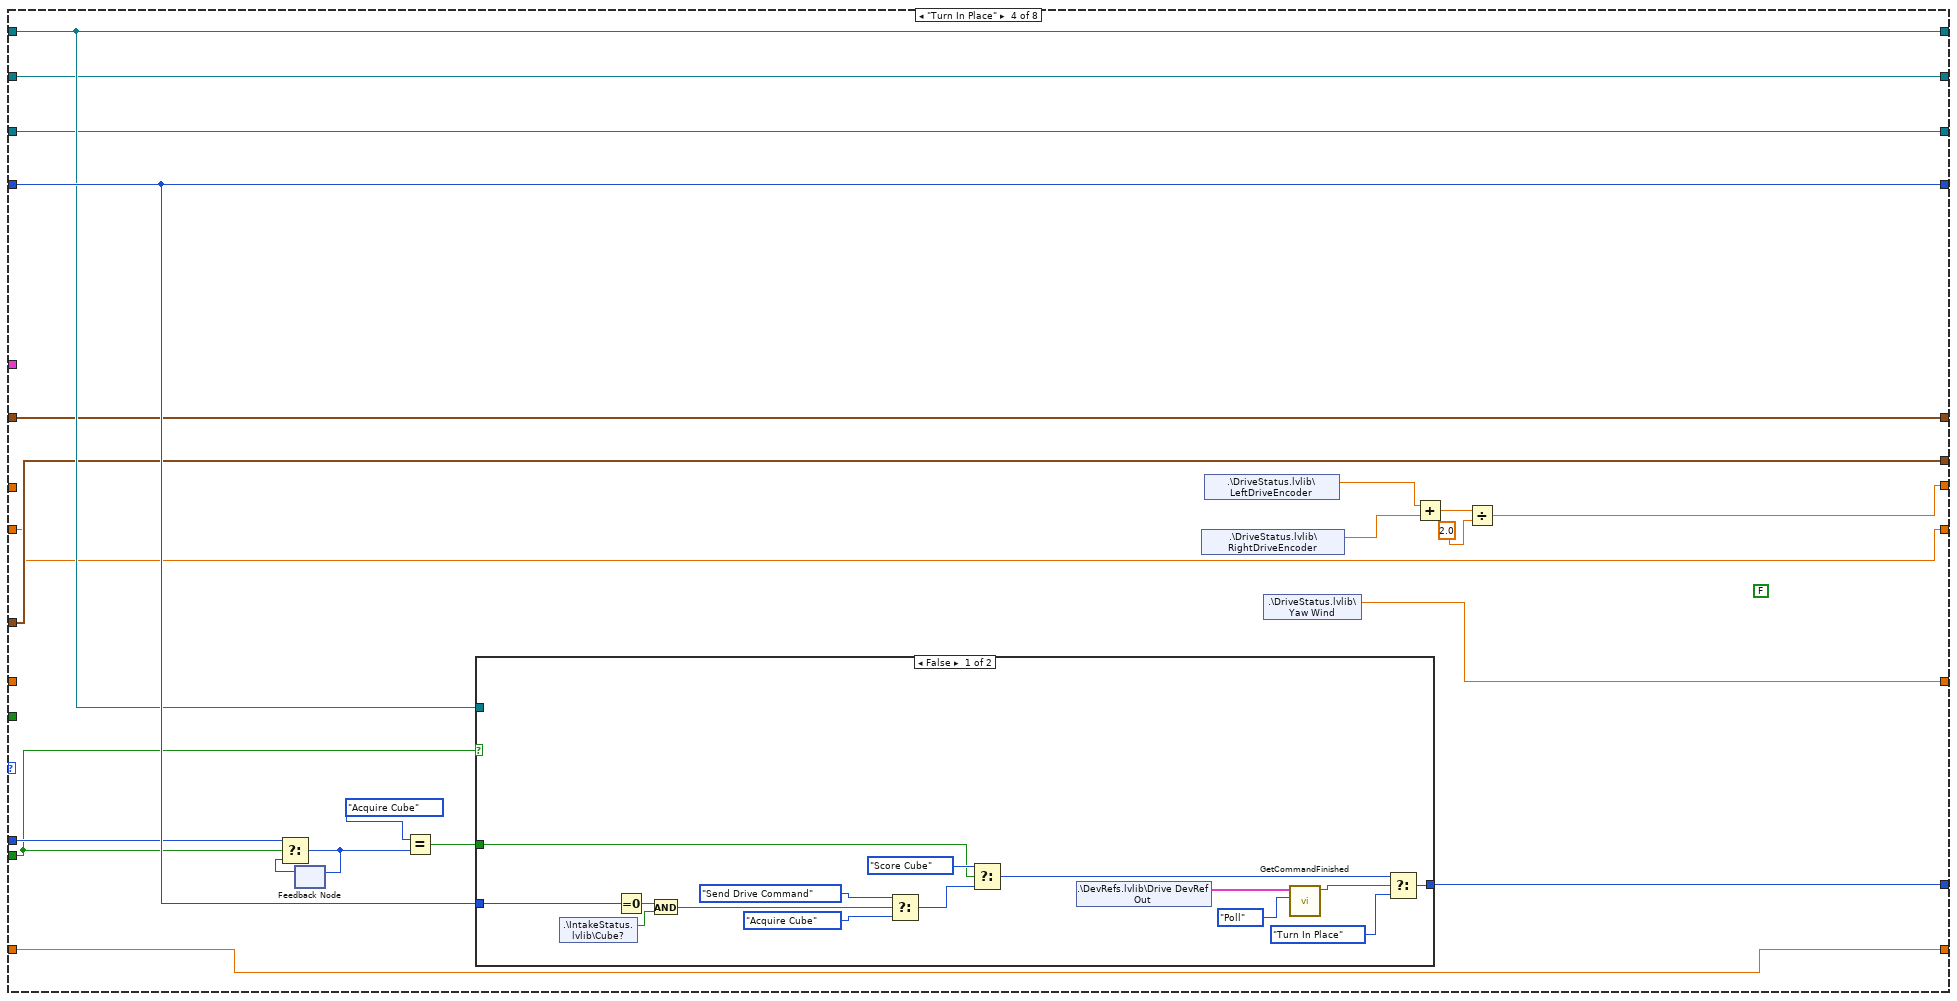
[diagram p13: hidden frame]
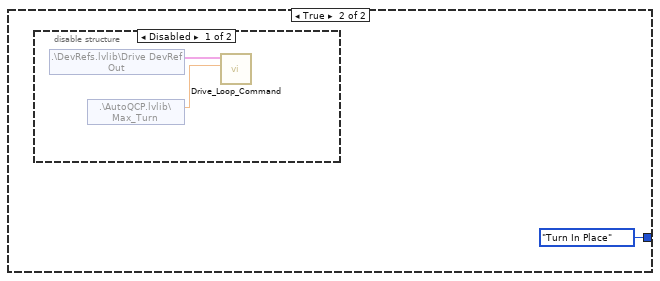
[diagram p14: hidden frame]
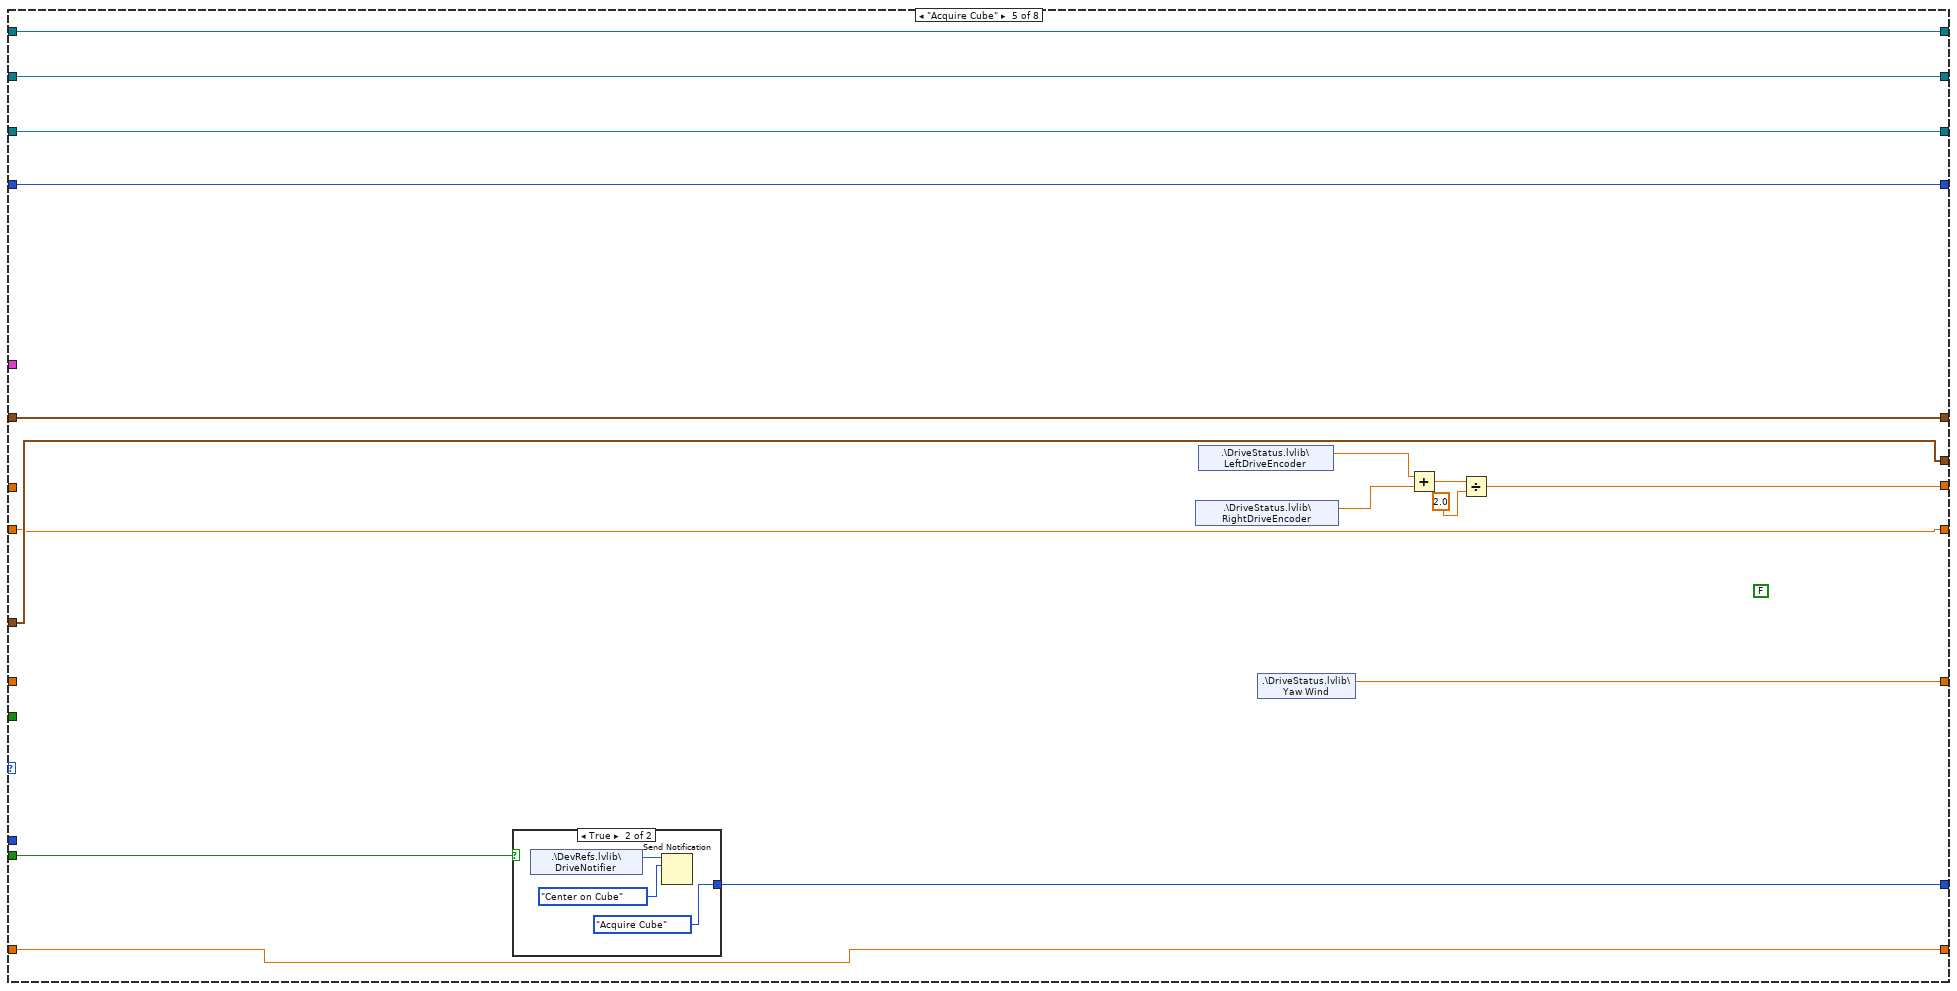
[diagram p16: hidden frame]
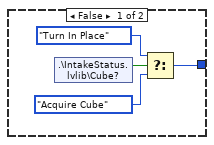
[diagram p17: hidden frame]
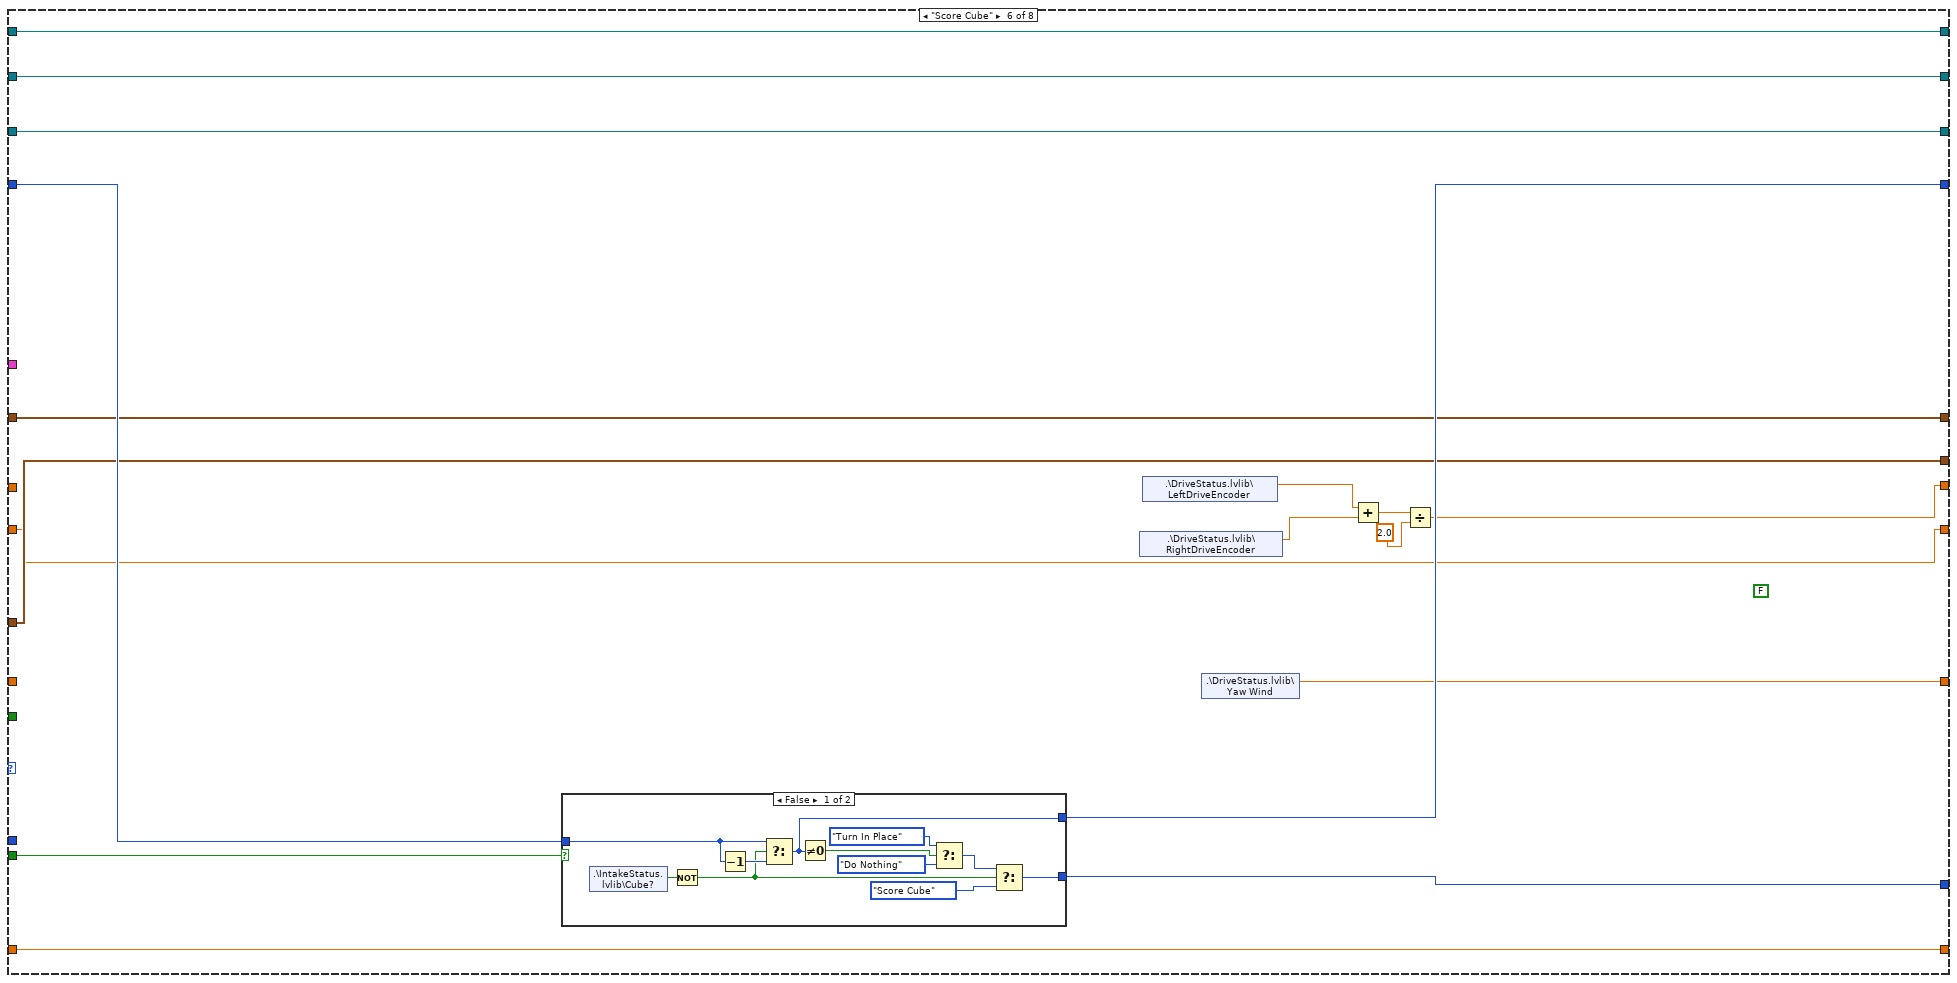
[diagram p18: hidden frame]
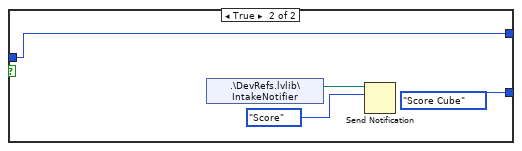
[diagram p19: hidden frame]
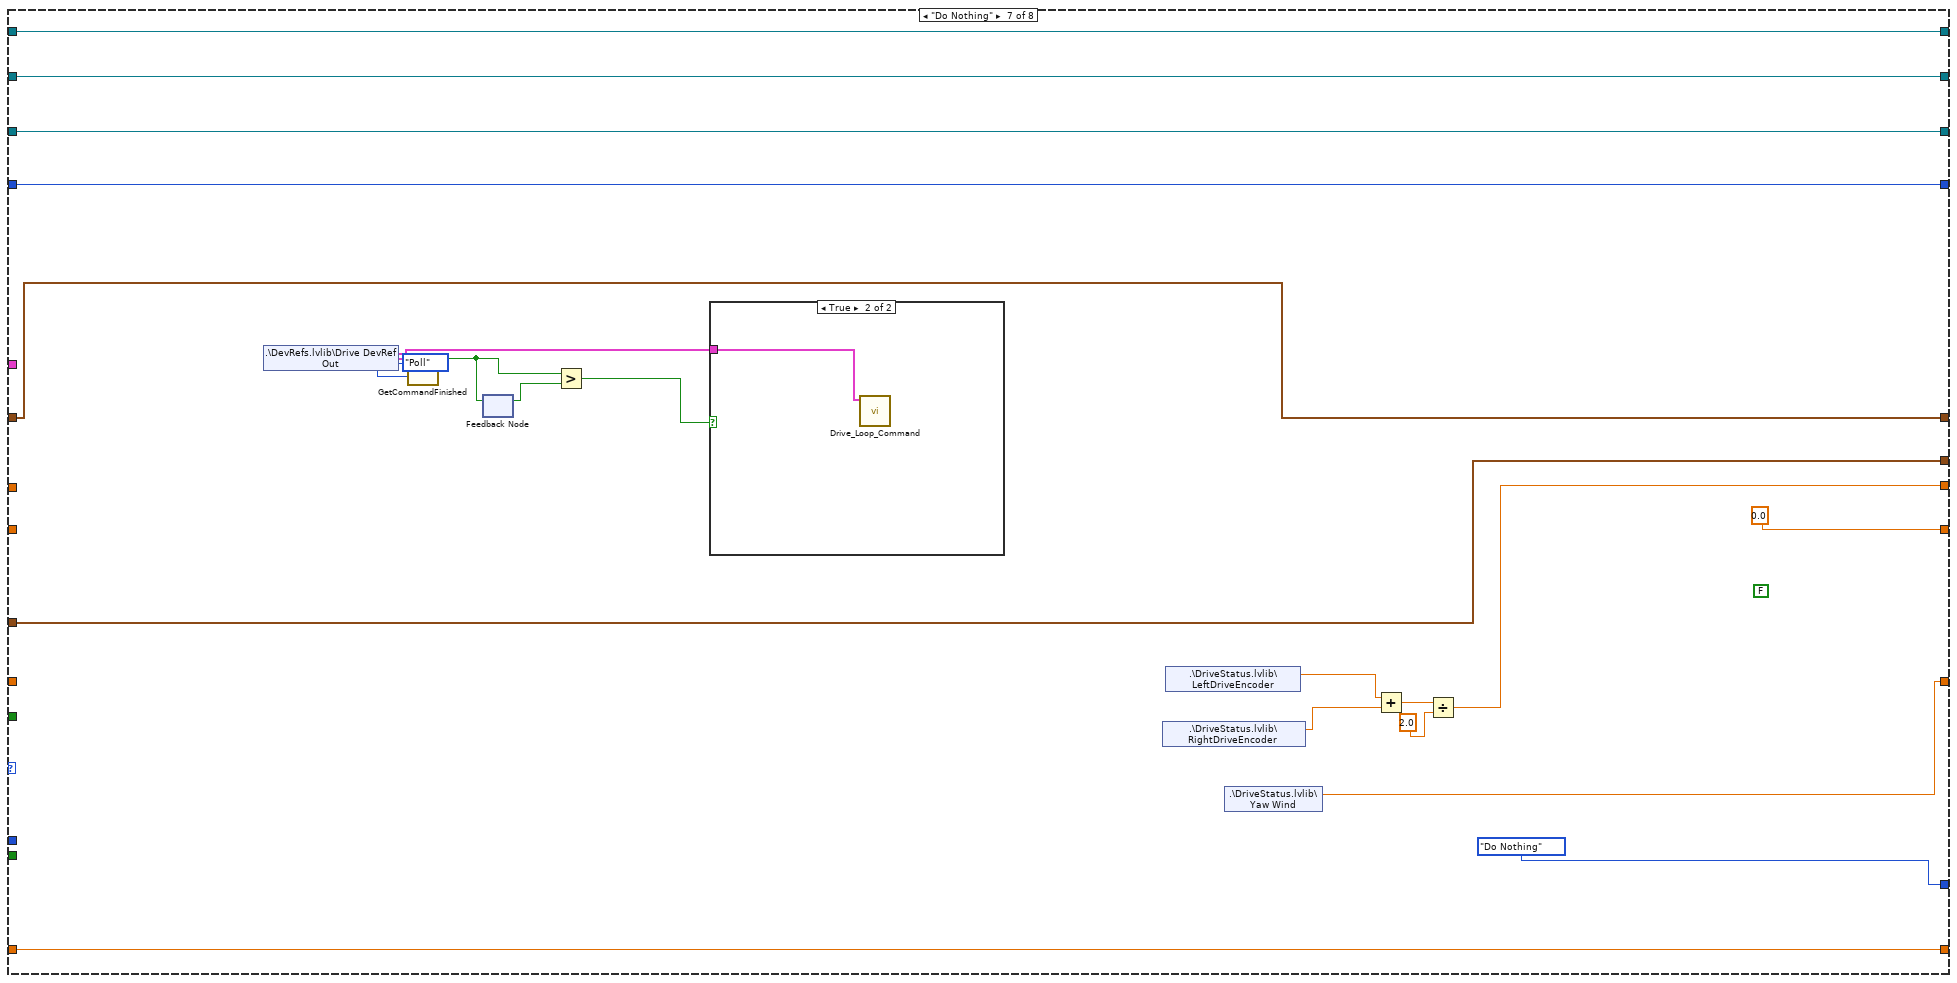
[diagram p20: hidden frame]
diagram:
  (unwired) enum16{"Switch_L", "Switch_R"}."Switch_L"
  # "Ref Time"
  # "right"
  # "left"
  # "encoder ref"
  # "# cubes to score"
  n1 = shared-variable ".\\DriveStatus.lvlib\\RightDriveEncoder"() -> (w6:dbl)  [unwired: 1 in, 1 out]
  n2 = shared-variable ".\\DriveStatus.lvlib\\LeftDriveEncoder"() -> (w5:dbl)  [unwired: 1 in, 1 out]
  n3 = Add(x=w5, y=w6) -> (x+y=w7:dbl)
  n4 = shared-variable ".\\DriveStatus.lvlib\\Yaw Wind"() -> (w3:dbl)  [unwired: 1 in, 1 out]
  n5 = Divide(x=w7, y=2.0) -> (x/y=w4:dbl)
  n6 = Obtain Queue(name (unnamed)="Turns", element data type=0.0) -> (queue out=w19:refnum<queue>)  [unwired: 3 in, 2 out]
  n7 = Obtain Queue(name (unnamed)="Splines", element data type=cluster{"X Points":dbl[], "Y Points":dbl[]} {"X Points"=[], "Y Points"=[]}) -> (queue out=w18:refnum<queue>)  [unwired: 3 in, 2 out]
  n8 = Obtain Queue(name (unnamed)="Elevator Heights", element data type=LiftCommands."Do  Nothing" ("notification")) -> (queue out=w17:refnum<queue>)  [unwired: 3 in, 2 out]
  n9 = call-poly <vilib>:"NT Read Value.vi"("Name"="Start_Delay") -> ("Numeric"=w10:dbl)  [unwired: 9 in, 1 out]
  n10 = node-c288(i64 50 ("Period")) -> (w23:T4)  [unwired: 3 in]
  n11 = timed-loop {
    timing: w23 -> [_]
    timing-out: [_] -> w22
    shift-right: [w51] -> _
    shift-left: AutoCommands."Delay" ("f") -> [w43]
    shift-right: [w50] -> _
    shift-left: 0 -> [w49]
    shift-right: [w40] -> _
    shift-left: w19 -> [w46]
    shift-right: [w39] -> _
    shift-left: w18 -> [w45]
    shift-right: [w38] -> _
    shift-left: w17 -> [w44]
    shift-right: [w41] -> _
    shift-left: w10 -> [w42]
    shift-right: [w37] -> _
    shift-left: _ -> [w35]
    shift-right: [w36] -> _
    shift-left: _ -> [w30]
    shift-right: [w34] -> _
    shift-left: w4 -> [w33]
    shift-right: [w31] -> _
    shift-left: w3 -> [w32]
    tunnel: cluster{"X Points":dbl[], "Y Points":dbl[]}[] [{"X Points"=[20.0, 70.0, 130.0], "Y Points"=[159.5, 200.0, 215.0]}, {"X Points"=[20.0, 70.0, 130.0], "Y Points"=[159.5, 140.0, 110.0]}] -> [w29]
    shift-right: [w28] -> _
    shift-left: _ -> [w27]
    stop <- _ stop-if-true
    n12 = node-c288() -> ()  [unwired: 1 in, 1 out]
    n13 = feedback #1(w43) -> (w47:T3)
    n14 = feedback-in #1(w43) -> ()
    n15 = call-poly <vilib>:"NT Read Value.vi"("Default Value"=FALSE, "Name"="Scale_First") -> ("Boolean"=w25:bool)  [unwired: 8 in, 1 out]
    n16 = Not Equal?(x=w43, y=w47) -> (x != y?=w48:bool)
    n17 = case shown="\"Move Lift\"" w43 {
      tunnel: [w79 w156 w227 w288 w321 w345 AutoCommands."Do Nothing" ("f") AutoCommands."Do Nothing" ("f")] -> w51
      tunnel: [w80 w180 w250 w287 w322 w344 w381 w404] -> w50
      tunnel: w49 -> [w82 w180 w250 w287 w322 w346 w381 w404]
      tunnel: w48 -> [w74 _ _ w282 w320 w343 _ _]
      tunnel: w47 -> [_ _ _ w283 _ _ _ _]
      tunnel: w46 -> [w71 w158 w246 w279 w318 w341 w379 w407]
      tunnel: w45 -> [w72 w176 w248 w278 w317 w340 w378 w406]
      tunnel: w44 -> [w70 w177 w247 w277 w316 w339 w377 w405]
      tunnel: w42 -> [w56 w178 w249 w280 w319 w342 w376 w403]
      tunnel: [w56 w178 w249 w280 w319 w342 w376 w403] -> w41
      tunnel: [w71 w158 w246 w279 w318 w341 w379 w407] -> w40
      tunnel: [w72 w176 w248 w278 w317 w340 w378 w406] -> w39
      tunnel: [w70 w177 w247 w277 w316 w339 w377 w405] -> w38
      tunnel: [w69 w165 w232 w276 w309 w338 w370 w391] -> w37
      tunnel: [w68 w164 w231 w275 w308 w337 w369 w390] -> w36
      tunnel: w35 -> [w69 _ w232 w276 w309 w338 w370 w391]
      tunnel: [w63 w131 w209 w270 w311 w332 w364 w385] -> w34
      tunnel: w33 -> [_ _ w209 _ _ _ _ _]
      tunnel: w32 -> [_ _ w236 _ _ _ _ _]
      tunnel: [w62 w132 w236 w269 w310 w331 w363 w384] -> w31
      tunnel: w30 -> [w68 _ w231 w275 w308 w337 w369 w390]
      tunnel: w29 -> [_ w142 _ _ _ _ _ _]
      tunnel: [0.0 w136 w214 w268 w307 w330 0.0 w383] -> w28
      tunnel: w27 -> [_ _ w214 w268 w307 w330 _ w383]
      tunnel: w25 -> [_ w130 w200 _ _ _ _ _]
      frame "Delay", Default {
        (unwired) FALSE
        # "Find real way to do this"
        # "Fixes problem where first call is only true the first iteration, thus causing us to never\nbe able to do a drive straight auto if there was any delay value other than 0 sec.\nWorks on the idea that the JK latch will set when the condition is met that we want\nto drive straight (the first iteration the delay state is run the entirity of auto) and\nwill reset when we enter delay a second time in auto. This is necessary because the \nboolean that determines if we are entering the state for the first time doesn't work\nthe first iteration of auto because our initial state is auto, the same state we are\ninitializing the feedback node to."
        # "Generate Points\nGenerate Turn angle Array\nGenerate eleveator heights"
        n18 = First Call?() -> (First Call?: T/F=w61:bool)
        n19 = case shown="True" w61 {
          tunnel: [w118 1] -> w80
          tunnel: w82 -> [w118 _]
          frame False {
          }
          frame True {
            n20 = call-poly <vilib>:"NT Read Value.vi"("Name"="Cubes_On_Switch") -> ("Numeric"=w122:dbl)  [unwired: 9 in, 1 out]
            n21 = call-poly <vilib>:"NT Read Value.vi"("Name"="Cubes_On_Scale") -> ("Numeric"=w121:dbl)  [unwired: 9 in, 1 out]
            n22 = Add(x=w122, y=w121) -> (x+y=w120:dbl)
            n23 = To Long Integer(number=w120) -> ()  [unwired: 1 out]
          }
        }
        n24 = disable-structure shown="Enabled" {
          disable-tunnel: w72 -> [w87 _]
          disable-tunnel: w71 -> [w86 _]
          disable-tunnel: w70 -> [w85 _]
          disable-tunnel: w61 -> [w84 _]
          disable-tunnel: [_ w108] -> w53
          frame Disabled {
            n25 = case shown="True" w84 {
              tunnel: w87 -> [_ w93]
              tunnel: w86 -> [_ w92]
              tunnel: w85 -> [_ w91]
              frame False {
              }
              frame True {
                n26 = call "StartPointToEndPoint.vi"() -> ("Points"=w95:T13[])  [unwired: 11 in]
                n27 = Array Size(array=w95) -> (size(s)=w94:i32)
                n28 = Decrement(x=w94) -> (x-1=w96:i32)
                n29 = for {
                  N: w96 -> [_]
                  tunnel: w95 -> [w105]
                  tunnel: w93 -> [w102]
                  tunnel: w92 -> [w101]
                  tunnel: w91 -> [w100]
                  tunnel: [w99] -> w90 mode=indexing
                  tunnel: [w98] -> w89 mode=indexing
                  tunnel: [w97] -> w88 mode=indexing
                  i -> [w106]
                  n30 = Decrement(x=w106) -> (x-1=w107:i32)
                  n31 = Index Array(array=w105, index #1=w106, index #2=w107) -> (element #1=w104:T13, element #2=w103:T13)
                  n32 = call "GetPathInfo.vi"("End Point"=w103, "Start Point"=w104) -> ("Elevator Command"=w97:T2, "Theta Final"=w98:dbl, "Points"=w99:cluster{"X Points":dbl[], "Y Points":dbl[]})  [unwired: 7 in]
                  n33 = Enqueue Element(queue=w102, element=w99) -> ()  [unwired: 2 in, 3 out]
                  n34 = Enqueue Element(queue=w101, element=w98) -> ()  [unwired: 2 in, 3 out]
                  n35 = Enqueue Element(queue=w100, element=w97) -> ()  [unwired: 2 in, 3 out]
                }
                "Init Points Queue" <- w90
                "Init Turns Queue" <- w89
                "Init Heights Queue" <- w88
              }
            }
          }
          frame Enabled {
            n36 = while {
              tunnel: [w109] -> w108
              stop <- w114 stop-if-true
              # "Game Data Acquisition Loop"
              n37 = call <vilib>:"WPI_DriverStationGame Specific Data.vi"() -> ("Game Specific Data"=w112:string)  [unwired: 11 in]
              n38 = shared-variable ".\\RobotSpecific.lvlib\\WaitGameDataTimeMs"() -> (w116:dbl)  [unwired: 1 in, 1 out]
              n39 = Wait (ms)(milliseconds to wait=u32 20) -> ()  [unwired: 1 out]
              n40 = shared-variable ".\\Match Data.lvlib\\GameData"(w112) -> ()  [unwired: 1 in, 1 out]
              n41 = String Length(string=w112) -> (length=w117:i32)
              n42 = Greater Or Equal To 0?(x=w117) -> (x >= 0?=w109:bool)
              n43 = First Call?() -> (First Call?: T/F=w115:bool)
              n44 = shared-variable ".\\Match Data.lvlib\\GameDataValid?"(w109) -> ()  [unwired: 1 in, 1 out]
              n45 = Not(x=w115) -> (.not. x?=w110:bool)
              n46 = call <userlib>:"Timer.vi"("Start"=w110, "Time (ms)"=w116) -> ("Time Expired?"=w113:bool)  [unwired: 6 in, 3 out]
              n47 = Or(x=w109, y=w113) -> (x .or. y?=w114:bool)
            }
          }
        }
        n48 = disable-structure shown="Disabled" {
          frame Disabled {
            n49 = call "Auto.vi"() -> ()  [unwired: 12 in]
          }
          frame Enabled {
          }
        }
        n50 = Multiply(x=w56, y=1000.0) -> (x*y=w58:dbl)
        n51 = Not(x=w61) -> (.not. x?=w59:bool)
        n52 = call <userlib>:"Timer.vi"("Start"=w59, "Time (ms)"=w58) -> ("Time Expired?"=w60:bool)  [unwired: 6 in, 3 out]
        n53 = Equal To 0?(x=w80) -> (x = 0?=w81:bool)
        n54 = And(x=w81, y=w59) -> (x .and. y?=w75:bool)
        n55 = call <userlib>:"JK_Latch.vi"("Reset"=w74, "Set"=w75) -> ("Q"=w73:bool)  [unwired: 5 in]
        n56 = shared-variable ".\\DriveStatus.lvlib\\RightDriveEncoder"() -> (w66:dbl)  [unwired: 1 in, 1 out]
        n57 = shared-variable ".\\DriveStatus.lvlib\\LeftDriveEncoder"() -> (w67:dbl)  [unwired: 1 in, 1 out]
        n58 = shared-variable ".\\DriveStatus.lvlib\\Yaw Wind"() -> (w62:dbl)  [unwired: 1 in, 1 out]
        n59 = Not(x=w53) -> (.not. x?=w54:bool)
        n60 = Or(x=w54, y=w73) -> (x .or. y?=w55:bool)
        n61 = Add(x=w67, y=w66) -> (x+y=w65:dbl)
        n62 = Divide(x=w65, y=2.0) -> (x/y=w63:dbl)
        n63 = Select(t=AutoCommands."Drive Straight", s=w55, f=AutoCommands."Send Drive Command") -> (s? t:f=w78:T3)
        n64 = Select(t=w78, s=w60, f=AutoCommands."Delay") -> (s? t:f=w79:T3)
      }
      frame "Send Drive Command" {
        n65 = shared-variable ".\\Match Data.lvlib\\GameData"() -> (w148:string)  [unwired: 1 in, 1 out]
        n66 = String Subset(string=w148, length (rest)=1 ("length (rest)")) -> (substring=w146:string)  [unwired: 1 in]
        n67 = To Upper Case(1:w146) -> (0:w145:string)
        n68 = shared-variable ".\\DriveStatus.lvlib\\Yaw Wind"() -> (w132:dbl)  [unwired: 1 in, 1 out]
        n69 = Index Array(array=w142) -> (element #1=w141:cluster{"X Points":dbl[], "Y Points":dbl[]}, element #2=w140:cluster{"X Points":dbl[], "Y Points":dbl[]})  [unwired: 2 in]
        n70 = Equal?(x="L", y=w145) -> (x = y?=w143:bool)
        n71 = Select(t=w141, s=w143, f=w140) -> (s? t:f=w139:cluster{"X Points":dbl[], "Y Points":dbl[]})
        n72 = Unbundle By Name(w139) -> ("X Points"=w125:dbl[], "Y Points"=w126:dbl[])
        n73 = disable-structure shown="Disabled" {
          disable-tunnel: w158 -> [w185 _]
          frame Disabled {
            n74 = Dequeue Element(queue=w185) -> ()  [unwired: 2 in, 4 out]
          }
          frame Enabled {
          }
        }
        n75 = Negate(x=w126) -> (-x=w133:dbl[])
        n76 = Select(t=w133, s=w130, f=w126) -> (s? t:f=w134:dbl[])
        n77 = Bundle By Name(cluster=T7 {"Absolute Theta initial"=0.0, "Absolute Theta Final"=0.0} ("Angle Info (Radians)"), "Absolute Theta initial"=0.0, "Absolute Theta Final"="Absolute Theta Final") -> (w174:T7)
        n78 = disable-structure shown="Disabled" {
          disable-tunnel: w176 -> [w184 _]
          frame Disabled {
            n79 = Dequeue Element(queue=w184) -> (element=w183:cluster{"X Points":dbl[], "Y Points":dbl[]})  [unwired: 2 in, 3 out]
            n80 = Unbundle By Name(w183) -> ()  [unwired: 2 out]
          }
          frame Enabled {
          }
        }
        n81 = Index Array(array=w134) -> (element=w149:dbl)  [unwired: 1 in]
        n82 = Index Array(array=w125) -> (element=w150:dbl)  [unwired: 1 in]
        n83 = Bundle(w150, w149) -> (w151:cluster{dbl, dbl})  [unwired: 1 in]
        n84 = call <userlib>:"Re-Origin.vi"("Transition"=w151, "Y"=w134, "X"=w125) -> ("Normalized Y"=w152:dbl[], "Normalized X"=w153:dbl[])  [unwired: 7 in]
        n85 = call <userlib>:"GenerateSpline.vi"("Amount of Time (s)"="Amount of Time (s)", "Number Of Samples"=500, "Limit of Orientation Change"="Limit of Orientation Change", "Angle Info (Radians)"=w174, "Y"=w152, "X"=w153) -> ("Verify Graph"=→"Auto Path Graph":cluster{"X":dbl, "Y":dbl}[], "Theta(arc length)"=w168:dbl[], "Arc Length"=w169:dbl[], "TimeStamp"=w167:dbl[])  [unwired: 2 in]
        n86 = Build Cluster Array(w167, w169) -> (w171:cluster{dbl, dbl}[])
        n87 = Build Cluster Array(w167, w168) -> (w170:cluster{dbl, dbl}[])
        n88 = Array Size(array=w167) -> (size(s)=w172:i32)
        n89 = for {
          N: "Pid Setpoints" -> [w198]
          tunnel: w172 -> [w196]
          tunnel: w171 -> [w190]
          tunnel: w170 -> [w189]
          tunnel: [w187] -> w165 mode=indexing
          tunnel: [w186] -> w164 mode=indexing
          i -> [w194]
          n90 = Reciprocal(x=w198) -> (1/x=w197:dbl)
          n91 = Increment(x=w194) -> (x+1=w193:i32)
          n92 = Multiply(x=w197, y=w196) -> (x*y=w195:dbl)
          n93 = Round Toward -Infinity(1:w195) -> (0:w192:dbl)
          n94 = Multiply(x=w192, y=w193) -> (x*y=w191:dbl)
          n95 = Decrement(x=w191) -> (x-1=w188:dbl)
          n96 = Index Array(array=w190, index=w188) -> (element=w187:cluster{dbl, dbl})
          n97 = Index Array(array=w189, index=w188) -> (element=w186:cluster{dbl, dbl})
        }
        n98 = shared-variable ".\\DriveStatus.lvlib\\RightDriveEncoder"() -> (w161:dbl)  [unwired: 1 in, 1 out]
        n99 = shared-variable ".\\DriveStatus.lvlib\\LeftDriveEncoder"() -> (w162:dbl)  [unwired: 1 in, 1 out]
        n100 = Not Equal To 0?(x=w180) -> (x != 0?=w181:bool)
        n101 = Select(t=AutoCommands."Move Lift", s=w181, f=AutoCommands."Do Nothing") -> (s? t:f=w156:T3)
        n102 = Add(x=w162, y=w161) -> (x+y=w160:dbl)
        n103 = Divide(x=w160, y=2.0) -> (x/y=w131:dbl)
        n104 = Decrement(x="Amount of Time (s)") -> (x-1=w128:dbl)
        n105 = Get Date/Time In Seconds() -> (seconds since 1Jan1904=w138:timestamp)
        n106 = Decrement(x=w128) -> (x-1=w129:dbl)
        n107 = Select(t=w129, s=w130, f=w128) -> (s? t:f=w127:dbl)
        n108 = To Double Precision Float(number=w138) -> (double precision float=w137:dbl)
        n109 = Add(x=w137, y=w127) -> (x+y=w136:dbl)
      }
      frame "Move Lift" {
        # "Also handles the waiting until spline has finished moving"
        n110 = Get Date/Time In Seconds() -> (seconds since 1Jan1904=w216:timestamp)
        n111 = To Double Precision Float(number=w216) -> (double precision float=w215:dbl)
        n112 = shared-variable ".\\DriveStatus.lvlib\\RightDriveEncoder"() -> (w244:dbl)  [unwired: 1 in, 1 out]
        n113 = shared-variable ".\\DriveStatus.lvlib\\LeftDriveEncoder"() -> (w245:dbl)  [unwired: 1 in, 1 out]
        n114 = Greater?(x=w215, y=w214) -> (0:w213:bool)
        n115 = shared-variable ".\\DriveStatus.lvlib\\Yaw Wind"() -> (w237:dbl)  [unwired: 1 in, 1 out]
        n116 = Add(x=w245, y=w244) -> (x+y=w243:dbl)
        n117 = Divide(x=w243, y=2.0) -> (x/y=w225:dbl)
        n118 = case shown="True" w213 {
          tunnel: w247 -> [_ _]
          frame False {
          }
          frame True {
            n119 = shared-variable ".\\DevRefs.lvlib\\LiftNotifier"() -> (w266:refnum<notifier>)  [unwired: 1 in, 1 out]
            n120 = Send Notification(notification=LiftCommands."To Switch", notifier=w266) -> ()  [unwired: 1 in, 2 out]
          }
        }
        n121 = Subtract(x=w237, y=w236) -> (x-y=w210:dbl)
        n122 = Subtract(x=w225, y=w209) -> (x-y=w208:dbl)
        n123 = call <vilib>:"PID Setpoint Profile.vi"("setpoint profile"=w231) -> ("profile complete?"=w230:bool, "setpoint"=w224:dbl)  [unwired: 5 in, 2 out]
        n124 = Negate(x=w208) -> (-x=w207:dbl)
        n125 = Negate(x=w210) -> (-x=w211:dbl)
        n126 = expression code="(x/pi)*180.0" "radians to degrees"(w224) -> (w217:dbl)
        n127 = Select(t=w207, s=w200, f=w208) -> (s? t:f=w206:dbl)
        n128 = Select(t=w211, s=w200, f=w210) -> (s? t:f=w212:dbl)
        n129 = call <vilib>:"PID Setpoint Profile.vi"("setpoint profile"=w232) -> ("profile complete?"=w218:bool, "setpoint"=w239:dbl)  [unwired: 5 in, 2 out]
        n130 = case shown="True" w218 {
          frame False {
          }
          frame True {
            n131 = flat-sequence {
              frame #0 {
                n132 = shared-variable ".\\DevRefs.lvlib\\BehindBackNotifier"() -> (w251:refnum<notifier>)  [unwired: 1 in, 1 out]
                n133 = Send Notification(notification=TRUE, notifier=w251) -> ()  [unwired: 1 in, 2 out]
              }
              frame #1 {
                n134 = Wait (ms)(milliseconds to wait=u32 1000) -> ()  [unwired: 1 out]
              }
              frame #2 {
                n135 = shared-variable ".\\Joystick.lvlib\\Button_LB"(TRUE ("Button_LB")) -> ()  [unwired: 1 in, 1 out]
              }
              frame #3 {
                n136 = Wait (ms)(milliseconds to wait=u32 1000) -> ()  [unwired: 1 out]
              }
              frame #4 {
                n137 = shared-variable ".\\DevRefs.lvlib\\BehindBackNotifier"() -> (w257:refnum<notifier>)  [unwired: 1 in, 1 out]
                n138 = shared-variable ".\\Joystick.lvlib\\Button_LB"(FALSE ("Button_LB")) -> ()  [unwired: 1 in, 1 out]
                n139 = Send Notification(notification=FALSE, notifier=w257) -> ()  [unwired: 1 in, 2 out]
              }
              frame #5 {
                n140 = Wait (ms)(milliseconds to wait=u32 1000) -> ()  [unwired: 1 out]
              }
              frame #6 {
                n141 = shared-variable ".\\DevRefs.lvlib\\LiftNotifier"() -> (w260:refnum<notifier>)  [unwired: 1 in, 1 out]
                n142 = Send Notification(notification=LiftCommands."To Switch", notifier=w260) -> ()  [unwired: 1 in, 2 out]
              }
              frame #7 {
                n143 = Wait (ms)(milliseconds to wait=u32 1000) -> ()  [unwired: 1 out]
              }
              frame #8 {
                n144 = shared-variable ".\\DevRefs.lvlib\\LiftNotifier"() -> (w264:refnum<notifier>)  [unwired: 1 in, 1 out]
                n145 = Send Notification(notification=LiftCommands."Home", notifier=w264) -> ()  [unwired: 1 in, 2 out]
              }
            }
          }
        }
        n146 = call-poly <vilib>:"PID.vi"("output range"="Speed Limit", "PID gains"="Speed Gains", "process variable"=w206, "setpoint"=w239) -> ("output"=w220:dbl)  [unwired: 6 in, 1 out]
        n147 = call-poly <vilib>:"PID.vi"("output range"="Steer Limit", "PID gains"="Steer Gains", "process variable"=w212, "setpoint"=w217) -> ("output"=w219:dbl)  [unwired: 6 in, 1 out]
        n148 = Bundle("setpoint"=w239, w206) -> (→"Arc Response":cluster{"setpoint":dbl, dbl})  [unwired: 1 in]
        n149 = Bundle("setpoint"=w217, w212) -> (→"Steer Response":cluster{"setpoint":dbl, dbl})  [unwired: 1 in]
        n150 = shared-variable ".\\DevRefs.lvlib\\Drive DevRef Out"() -> (w223:T24)  [unwired: 1 in, 1 out]
        n151 = Add(x="Throttle Feed Fwd", y=w220) -> (x+y=w201:dbl)
        n152 = Negate(x=w219) -> (-x=w205:dbl)
        n153 = Negate(x=w201) -> (-x=w202:dbl)
        n154 = Negate(x=w205) -> (-x=w204:dbl)
        n155 = Select(t=w204, s=w200, f=w205) -> (s? t:f=w203:dbl)
        "Steer Cmd" <- w203
        n156 = Select(t=w202, s=w200, f=w201) -> (s? t:f=w199:dbl)
        "Throttle Cmd" <- w199
        n157 = call-poly <userlib>:"Drive_Loop_Command.vi"("Wheel"=w203, "Throttle"=w199, "Drive Loop Cluster"=w223) -> ("error out"=w222:errorcluster)  [unwired: 8 in]
        n158 = And(x=w218, y=w230) -> (x .and. y?=w229:bool)
        n159 = case shown="True" w218 {
          tunnel: w223 -> [_ w267]
          tunnel: w222 -> [_ _]
          frame False {
          }
          frame True {
            n160 = call-poly <userlib>:"Drive_Loop_Command.vi"("Drive Loop Cluster"=w267) -> ()  [unwired: 11 in]
          }
        }
        n161 = Select(t=AutoCommands."Turn In Place" ("f"), s=w229, f=AutoCommands."Move Lift") -> (s? t:f=w227:T3)
      }
      frame "Turn In Place" {
        (unwired) FALSE
        n162 = feedback #2() -> (w284:T3)  [unwired: 1 in]
        n163 = Select(t=w283, s=w282, f=w284) -> (s? t:f=w286:T3)
        n164 = feedback-in #2(w286) -> ()
        n165 = Equal?(x=AutoCommands."Acquire Cube" ("f"), y=w286) -> (x = y?=w281:bool)
        n166 = case shown="False" w282 {
          tunnel: [w291 AutoCommands."Turn In Place" ("f")] -> w288
          tunnel: w287 -> [w290 _]
          tunnel: w279 -> [_ _]
          tunnel: w281 -> [w289 _]
          frame False {
            n167 = shared-variable ".\\IntakeStatus.lvlib\\Cube?"() -> (w293:bool)  [unwired: 1 in, 1 out]
            n168 = Equal To 0?(x=w290) -> (x = 0?=w303:bool)
            n169 = And(x=w303, y=w293) -> (x .and. y?=w302:bool)
            n170 = Select(t=AutoCommands."Send Drive Command" ("f"), s=w302, f=AutoCommands."Acquire Cube") -> (s? t:f=w292:T3)
            n171 = Select(t=AutoCommands."Score Cube", s=w289, f=w292) -> (s? t:f=w297:T3)
            n172 = shared-variable ".\\DevRefs.lvlib\\Drive DevRef Out"() -> (w300:T24)  [unwired: 1 in, 1 out]
            n173 = call <userlib>:"GetCommandFinished.vi"("Type"=CmdFinishedTypes."Poll", "DriveDevRefIn"=w300) -> ("Finished?"=w299:bool)  [unwired: 8 in, 1 out]
            n174 = Select(t=w297, s=w299, f=AutoCommands."Turn In Place") -> (s? t:f=w291:T3)
          }
          frame True {
            n175 = disable-structure shown="Disabled" {
              frame Disabled {
                n176 = shared-variable ".\\DevRefs.lvlib\\Drive DevRef Out"() -> (w306:T24)  [unwired: 1 in, 1 out]
                n177 = shared-variable ".\\AutoQCP.lvlib\\Max_Turn"() -> (w305:dbl)  [unwired: 1 in, 1 out]
                n178 = call-poly <userlib>:"Drive_Loop_Command.vi"("Max Power"=w305, "Drive Loop Cluster"=w306) -> ()  [unwired: 9 in, 1 out]
              }
              frame Enabled {
              }
            }
          }
        }
        n179 = shared-variable ".\\DriveStatus.lvlib\\RightDriveEncoder"() -> (w273:dbl)  [unwired: 1 in, 1 out]
        n180 = shared-variable ".\\DriveStatus.lvlib\\LeftDriveEncoder"() -> (w274:dbl)  [unwired: 1 in, 1 out]
        n181 = shared-variable ".\\DriveStatus.lvlib\\Yaw Wind"() -> (w269:dbl)  [unwired: 1 in, 1 out]
        n182 = Add(x=w274, y=w273) -> (x+y=w272:dbl)
        n183 = Divide(x=w272, y=2.0) -> (x/y=w270:dbl)
      }
      frame "Acquire Cube" {
        (unwired) FALSE
        n184 = case shown="True" w320 {
          tunnel: [w323 AutoCommands."Acquire Cube" ("f")] -> w321
          frame False {
            n185 = shared-variable ".\\IntakeStatus.lvlib\\Cube?"() -> (w326:bool)  [unwired: 1 in, 1 out]
            n186 = Select(t=AutoCommands."Turn In Place" ("f"), s=w326, f=AutoCommands."Acquire Cube") -> (s? t:f=w323:T3)
          }
          frame True {
            n187 = shared-variable ".\\DevRefs.lvlib\\DriveNotifier"() -> (w328:refnum<notifier>)  [unwired: 1 in, 1 out]
            n188 = Send Notification(notification=DriveCommands."Center on Cube" ("Enum"), notifier=w328) -> ()  [unwired: 1 in, 2 out]
          }
        }
        n189 = shared-variable ".\\DriveStatus.lvlib\\RightDriveEncoder"() -> (w314:dbl)  [unwired: 1 in, 1 out]
        n190 = shared-variable ".\\DriveStatus.lvlib\\LeftDriveEncoder"() -> (w315:dbl)  [unwired: 1 in, 1 out]
        n191 = shared-variable ".\\DriveStatus.lvlib\\Yaw Wind"() -> (w310:dbl)  [unwired: 1 in, 1 out]
        n192 = Add(x=w315, y=w314) -> (x+y=w313:dbl)
        n193 = Divide(x=w313, y=2.0) -> (x/y=w311:dbl)
      }
      frame "Score Cube" {
        (unwired) FALSE
        n194 = case shown="False" w343 {
          tunnel: w346 -> [w351 w361]
          tunnel: [w350 AutoCommands."Score Cube" ("f")] -> w345
          tunnel: [w349 w361] -> w344
          frame False {
            n195 = shared-variable ".\\IntakeStatus.lvlib\\Cube?"() -> (w348:bool)  [unwired: 1 in, 1 out]
            n196 = Not(x=w348) -> (.not. x?=w347:bool)
            n197 = Decrement(x=w351) -> (x-1=w354:i32)
            n198 = Select(t=w351, s=w347, f=w354) -> (s? t:f=w349:i32)
            n199 = Not Equal To 0?(x=w349) -> (x != 0?=w357:bool)
            n200 = Select(t=AutoCommands."Turn In Place" ("f"), s=w357, f=AutoCommands."Do Nothing") -> (s? t:f=w355:T3)
            n201 = Select(t=w355, s=w347, f=AutoCommands."Score Cube") -> (s? t:f=w350:T3)
          }
          frame True {
            n202 = shared-variable ".\\DevRefs.lvlib\\IntakeNotifier"() -> (w359:refnum<notifier>)  [unwired: 1 in, 1 out]
            n203 = Send Notification(notification=IntakeCommands."Score", notifier=w359) -> ()  [unwired: 1 in, 2 out]
          }
        }
        n204 = shared-variable ".\\DriveStatus.lvlib\\RightDriveEncoder"() -> (w335:dbl)  [unwired: 1 in, 1 out]
        n205 = shared-variable ".\\DriveStatus.lvlib\\LeftDriveEncoder"() -> (w336:dbl)  [unwired: 1 in, 1 out]
        n206 = shared-variable ".\\DriveStatus.lvlib\\Yaw Wind"() -> (w331:dbl)  [unwired: 1 in, 1 out]
        n207 = Add(x=w336, y=w335) -> (x+y=w334:dbl)
        n208 = Divide(x=w334, y=2.0) -> (x/y=w332:dbl)
      }
      frame "Do Nothing" {
        (unwired) FALSE
        n209 = shared-variable ".\\DevRefs.lvlib\\Drive DevRef Out"() -> (w371:T24)  [unwired: 1 in, 1 out]
        n210 = call <userlib>:"GetCommandFinished.vi"("Type"=CmdFinishedTypes."Poll", "DriveDevRefIn"=w371) -> ("Finished?"=w374:bool)  [unwired: 8 in, 1 out]
        n211 = feedback-in #3(w374) -> ()
        n212 = feedback #3() -> (w373:bool)  [unwired: 1 in]
        n213 = Greater?(x=w374, y=w373) -> (0:w372:bool)
        n214 = case shown="True" w372 {
          tunnel: w371 -> [_ w382]
          frame False {
          }
          frame True {
            n215 = call-poly <userlib>:"Drive_Loop_Command.vi"("Drive Loop Cluster"=w382) -> ()  [unwired: 11 in]
          }
        }
        n216 = shared-variable ".\\DriveStatus.lvlib\\RightDriveEncoder"() -> (w367:dbl)  [unwired: 1 in, 1 out]
        n217 = shared-variable ".\\DriveStatus.lvlib\\LeftDriveEncoder"() -> (w368:dbl)  [unwired: 1 in, 1 out]
        n218 = shared-variable ".\\DriveStatus.lvlib\\Yaw Wind"() -> (w363:dbl)  [unwired: 1 in, 1 out]
        n219 = Add(x=w368, y=w367) -> (x+y=w366:dbl)
        n220 = Divide(x=w366, y=2.0) -> (x/y=w364:dbl)
      }
      frame "Drive Straight" {
        (unwired) FALSE
        w393 = 3.0 ("Distance.Upper Error Bound")
        n221 = shared-variable ".\\DevRefs.lvlib\\Drive DevRef Out"() -> (w395:T24)  [unwired: 1 in, 1 out]
        n222 = shared-variable ".\\DriveStatus.lvlib\\RightDriveEncoder"() -> (w388:dbl)  [unwired: 1 in, 1 out]
        n223 = shared-variable ".\\DriveStatus.lvlib\\LeftDriveEncoder"() -> (w389:dbl)  [unwired: 1 in, 1 out]
        n224 = call-poly <userlib>:"Drive_Loop_Command.vi"("Max Forward Power"=0.7, "Absolute Angle?"=FALSE, "Absolute Distance?"=FALSE, "Angle"=0.0, "Max Turn Power"=0.7, "Distance"=95.0, "Drive Loop Cluster"=w395) -> ()  [unwired: 4 in, 1 out]
        n225 = shared-variable ".\\DriveStatus.lvlib\\Yaw Wind"() -> (w384:dbl)  [unwired: 1 in, 1 out]
        n226 = Bundle By Name(cluster=T11 {"Distance"={"Upper Error Bound"=0.0, "Lower Error Bound"=0.0}, "Yaw"={"Upper Error Bound"=0.0, "Lower Error Bound"=0.0}} ("Tolerance Settings"), "Distance.Upper Error Bound"=w393, "Distance.Lower Error Bound"=w393) -> (w392:T11)
        n227 = Add(x=w389, y=w388) -> (x+y=w387:dbl)
        n228 = Divide(x=w387, y=2.0) -> (x/y=w385:dbl)
        n229 = call <userlib>:"Drive_Update_Tolerance.vi"("Tolerance Settings"=w392, "Drive DevRef In"=w395) -> ()  [unwired: 10 in]
      }
    }
    n230 = node-c288() -> ()  [unwired: 1 in, 1 out]
  }
  n231 = while {
    stop <- w415 stop-if-true
    # "Game Data Acquisition Loop"
    n232 = call <vilib>:"WPI_DriverStationGame Specific Data.vi"() -> ("Game Specific Data"=w413:string)  [unwired: 11 in]
    n233 = shared-variable ".\\RobotSpecific.lvlib\\WaitGameDataTimeMs"() -> (w417:dbl)  [unwired: 1 in, 1 out]
    n234 = Wait (ms)(milliseconds to wait=u32 20) -> ()  [unwired: 1 out]
    n235 = shared-variable ".\\Match Data.lvlib\\GameData"(w413) -> ()  [unwired: 1 in, 1 out]
    n236 = String Length(string=w413) -> (length=w418:i32)
    n237 = Greater Or Equal To 0?(x=w418) -> (x >= 0?=w412:bool)
    n238 = First Call?() -> (First Call?: T/F=w416:bool)
    n239 = shared-variable ".\\Match Data.lvlib\\GameDataValid?"(w412) -> ()  [unwired: 1 in, 1 out]
    n240 = Not(x=w416) -> (.not. x?=w410:bool)
    n241 = call <userlib>:"Timer.vi"("Start"=w410, "Time (ms)"=w417) -> ("Time Expired?"=w414:bool)  [unwired: 6 in, 3 out]
    n242 = Or(x=w412, y=w414) -> (x .or. y?=w415:bool)
  }
  n243 = node-c288(w22) -> ()  [unwired: 1 out]
